vi "Chart.vi"() -> ()   [LabVIEW 2012]
uses:
  <vilib>/Utility/error.llb/DialogType.ctl
  <vilib>/Platform/TimedLoop/XDataNode/timing_clust.ctl
  <vilib>/Platform/TimedLoop/XDataNode/nitl_modes.ctl
  <vilib>/Platform/TimedLoop/XDataNode/wakeup.ctl
  <vilib>/Utility/error.llb/whitespace.ctl
  <vilib>/printing/EasyPrintingControls.llb/contents.ctl
  <vilib>/printing/EasyPrintingControls.llb/custom_contents_options.ctl
  <vilib>/printing/EasyPrintingControls.llb/list_which_controls.ctl
  <vilib>/printing/EasyPrintingControls.llb/layout_options.ctl
  <vilib>/printing/EasyPrintingControls.llb/orientation.ctl
  <vilib>/printing/EasyPrintingControls.llb/panel_scaling_for_page.ctl
  <vilib>/printing/EasyPrintingControls.llb/margins.ctl
  <vilib>/printing/EasyPrintingControls.llb/margin_values.ctl
  <vilib>/printing/EasyPrintingControls.llb/measurement_system.ctl
  <vilib>/printing/EasyPrintingControls.llb/printer_options.ctl
  <vilib>/printing/EasyPrintingControls.llb/printing_method.ctl
  <vilib>/printing/EasyPrintingControls.llb/color_or_monochrome.ctl
  <vilib>/printing/EasyPrintingControls.llb/page_header_options.ctl
  <vilib>/printing/EasyPrintingControls.llb/page_headers.ctl
  <vilib>/printing/EasyPrintingControls.llb/page_header_content_options.ctl
  <vilib>/DAQmx/read.llb/DAQmx Read (Analog 1D Wfm NChan NSamp).vi
  <vilib>/DAQmx/configure/timing.llb/DAQmx Timing (Sample Clock).vi
  <vilib>/DAQmx/create/channels.llb/DAQmx Create Channel (AI-Voltage-Basic).vi
  <vilib>/DAQmx/miscellaneous.llb/DAQmx Fill In Error Info.vi
  <vilib>/printing/EasyPrinting.llb/Easy Print VI Panel or Documentation (path).vi
  <vilib>/Platform/TimedLoop/XDataNode/XDataNode.xnode
  <vilib>/Platform/TimedLoop/XDataNode/XDNodeRunTimeDep.lvlib
  <resource>/objmgr/daqmx.rc
  <vilib>/Utility/NIReport.llb/NI_ReportGenerationCore.lvlib
panel:
  in  "Reset":bool
  in  "stop":bool
  in  "Tab Control":T1(tab)
  in  "Print1":bool
  in  "Capture1":bool
  in  "Samples Per Second":dbl(knob)=1.0 min=1.0 max=10.0 step=1.0 scale=1.0..10.0
  out "Waveform Chart1":waveform(dbl)(graph)
  in  "Clear1":bool
  in  "Save1":bool
  in  "Samples box1":bool
  in  "Title1":bool
  in  "Print12":bool
  out "Waveform Chart":dynamicdata(graph)
  in  "Capture12":bool
  in  "Clear12":bool
  in  "Save12":bool
  in  "Title12":bool
  in  "Samples Per Second":dbl(knob)=1.0 min=1.0 max=10.0 step=1.0 scale=1.0..10.0
  in  "Samples box12":bool
  in  "Print123":bool
  in  "Capture123":bool
  in  "Samples Per Second":dbl(knob)=1.0 min=1.0 max=10.0 step=1.0 scale=1.0..10.0
  out "Waveform Chart123":dynamicdata(graph)
  in  "Clear123":bool
  in  "Save123":bool
  in  "Samples box123":bool
  in  "Title123":bool
  in  "Print1234":bool
  in  "Capture1234":bool
  in  "Samples Per Second":dbl(knob)=1.0 min=1.0 max=10.0 step=1.0 scale=1.0..10.0
  in  "Save1234":bool
  in  "Samples box1234":bool
  in  "Title1234":bool
  out "Waveform Chart1234":dynamicdata(graph)
  in  "Clear1234":bool
  in  "Print1v2":bool
  out "XY Graph":cluster{"Y":dbl[], "Y":dbl[]}[](graph)
  in  "Title1v2":bool
  in  "Save1v2":bool
  in  "Clear1v2":bool
  in  "Samples Per Second":dbl(knob)=1.0 min=1.0 max=10.0 step=1.0 scale=1.0..10.0
  in  "Capture1v2":bool
  in  "Samples box1v2":bool
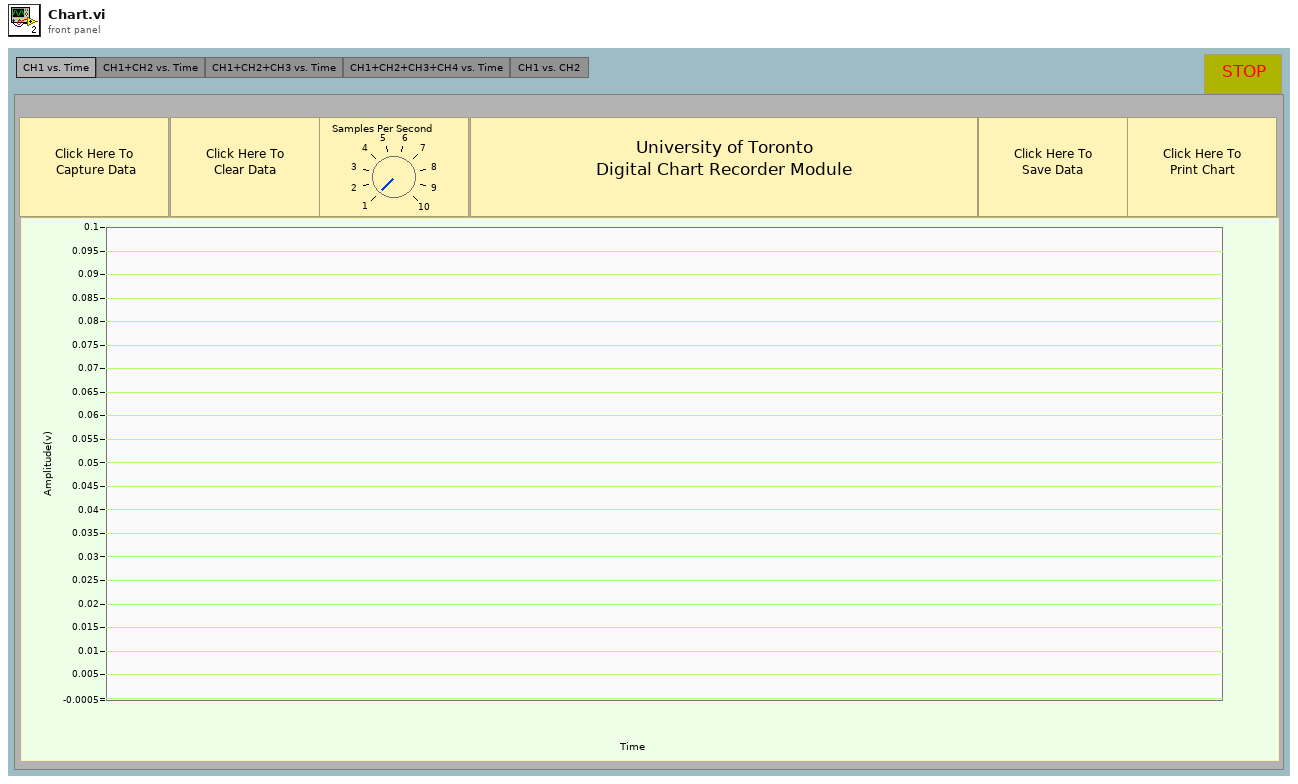
[diagram p1: front panel]
types:
  T1 = enum32{"CH1 vs. Time", "CH1+CH2 vs. Time", "CH1+CH2+CH3 vs. Time", "CH1+CH2+CH3+CH4 vs. Time", "CH1 vs. CH2 "}
  T2 = enum8{"Enabled", "Disabled", "Disabled and Grayed Out"}
  T3 = enum32{"CH1 vs. Time", "CH1+CH2 vs. Time", "CH1+CH2+CH3 vs. Time", "CH1+CH2+CH3+CH4 vs. Time", "CH1 vs. CH2  "}
  T4 = typedef "XDNodeRunTimeDep.lvlib/timing_clust.ctl" = cluster{"Expected End [f-1]":u64, "Actual End [f-1]":u64, "Finished Late? [f-1]":bool, "Expected End [i-1]":u64, "Actual End [i-1]":u64, "Finished Late? [i-1]":bool, "Expected Start [i]":u64, "Actual Start [i]":u64, "Expected Start [f]":u64, "Actual Start [f]":u64, "Source Name":string, "Structure Name":string, "Period":i64, "Deadline":i64, "Offset":i64, "Start":i64, "Priority":i32, "Timeout":i32, "Mode":T5, "Wakeup Reason":T6, "Error":errorcluster, "Source Type":string, "Secondary Source Type":string, "Global End Time":u64, "Global Start Time":u64, "Frame Duration":u64, "Iteration Duration":u64, "Assigned CPU":i32, "I/O Scan Engine Mode":u32}
  T5 = typedef "XDNodeRunTimeDep.lvlib/nitl_modes.ctl" = enum32{"No Change", "Process missed periods, maintain original phase", "Discard missed periods, maintain original phase", "Process missed periods, ignore original phase", "Discard missed periods, ignore original phase"}
  T6 = typedef "XDNodeRunTimeDep.lvlib/wakeup.ctl" = enum32{"Normal", "Aborted", "Asynchronous wakeup", "Timing source error", "Timed loop error", "Timeout"}
  T7 = enum16{"open", "replace", "create", "open or create", "replace or create", "replace or create with confirmation"}
  T8 = typedef "NI_ReportGenerationCore.lvlib/layout_options.ctl" = cluster{"orientation (unchanged)":T9, "panel scaling for page (unchanged)":T10, "margins":T11, "printer options":T14, "page header options":T17}
  T9 = typedef "NI_ReportGenerationCore.lvlib/orientation.ctl" = u16
  T10 = typedef "NI_ReportGenerationCore.lvlib/panel_scaling_for_page.ctl" = u16
  T11 = typedef "NI_ReportGenerationCore.lvlib/margins.ctl" = cluster{"override VI margins (false)":bool, "margins (1.00)":T12, "measurement system (default)":T13}
  T12 = typedef "NI_ReportGenerationCore.lvlib/margin_values.ctl" = cluster{"top":dbl, "left":dbl, "right":dbl, "bottom":dbl}
  T13 = typedef "NI_ReportGenerationCore.lvlib/measurement_system.ctl" = u16
  T14 = typedef "NI_ReportGenerationCore.lvlib/printer_options.ctl" = cluster{"destination printer name (current)":string, "printing method (unchanged)":T15, "color or monochrome (unchanged)":T16}
  T15 = typedef "NI_ReportGenerationCore.lvlib/printing_method.ctl" = u16
  T16 = typedef "NI_ReportGenerationCore.lvlib/color_or_monochrome.ctl" = u16
  T17 = typedef "NI_ReportGenerationCore.lvlib/page_header_options.ctl" = cluster{"page headers (unchanged)":T18, "page header content options":T19}
  T18 = typedef "NI_ReportGenerationCore.lvlib/page_headers.ctl" = u16
  T19 = typedef "NI_ReportGenerationCore.lvlib/page_header_content_options.ctl" = cluster{"Include VI Name":bool, "Include VI Path":bool, "Include Last Modification Date":bool, "Include Date Printed":bool, "Include Page Number":bool, "Include VI Icon":bool}
  T20 = typedef "NI_ReportGenerationCore.lvlib/custom_contents_options.ctl" = cluster{"include VI connector and icon":bool, "include VI description":bool, "include front panel":bool, "surround front panel with border":bool, "list of controls options":cluster{"include list of controls":bool, "list which controls?":T21, "include control descriptions?":bool, "include control data types?":bool}, "block diagram options":cluster{"include block diagram":bool, "hidden frames":bool, "ordered (repeat from higher level if nested)":bool}, "include VI hierarchy":bool, "include list of subVIs":bool, "include VI history":bool, "include Express VI configuration information":bool}
  T21 = typedef "NI_ReportGenerationCore.lvlib/list_which_controls.ctl" = u16
  T22 = typedef "DialogType.ctl" = u16
  T23 = typedef "whitespace.ctl" = u16
  T24 = typedef "NI_ReportGenerationCore.lvlib/contents.ctl" = u16
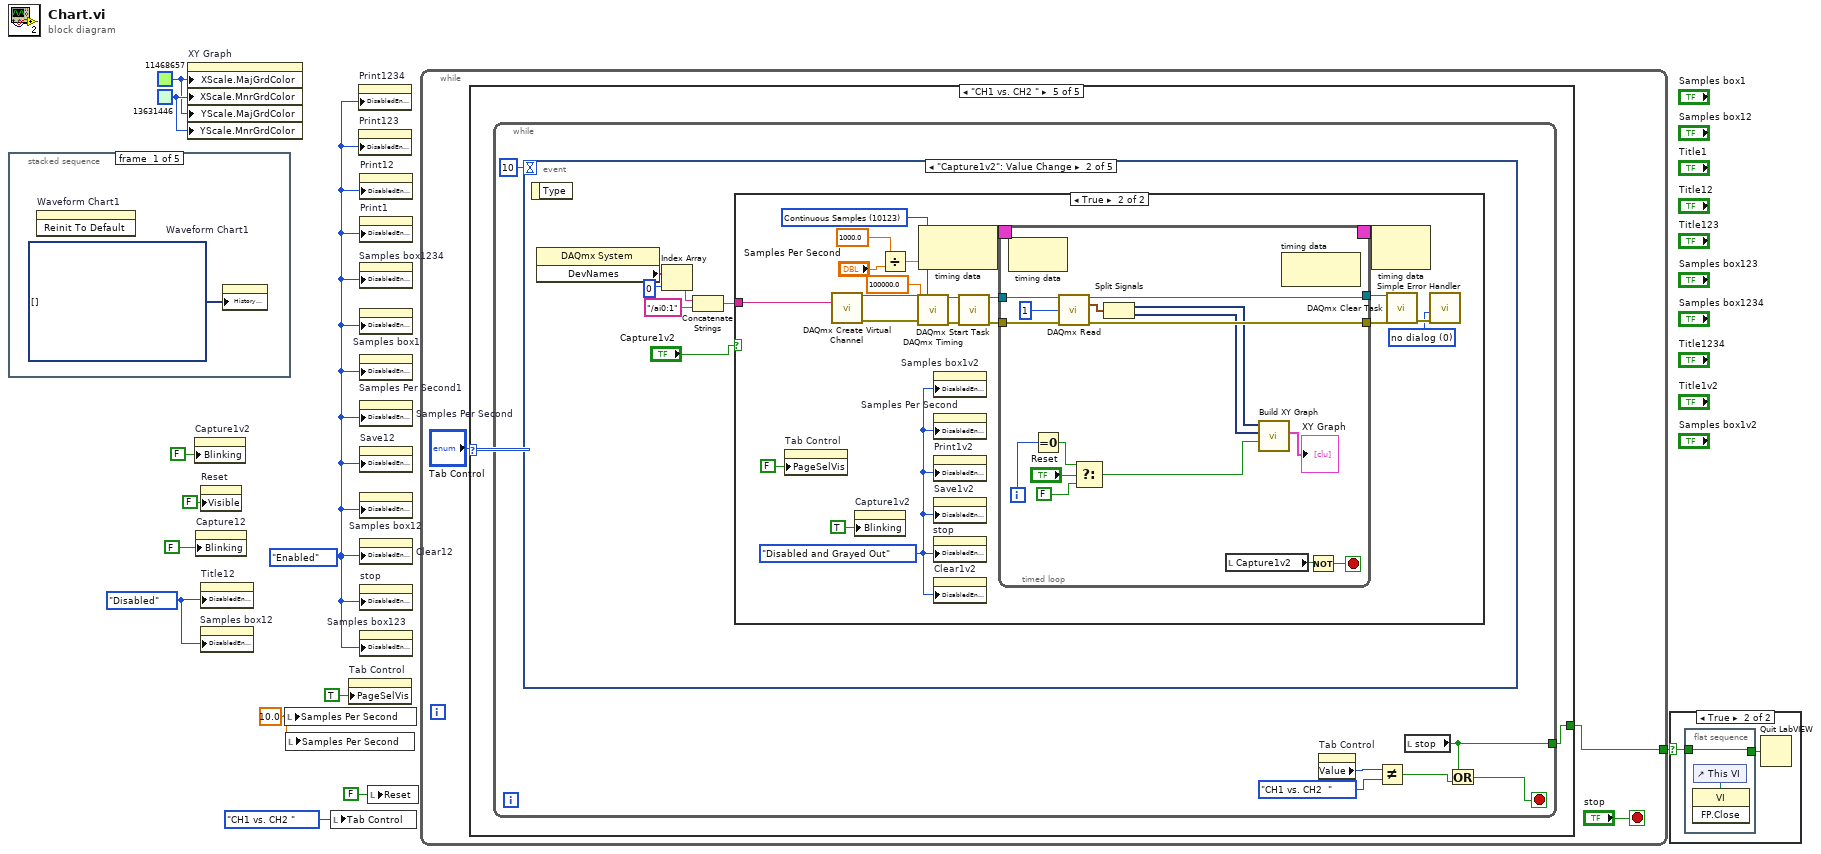
[diagram p0: block diagram]
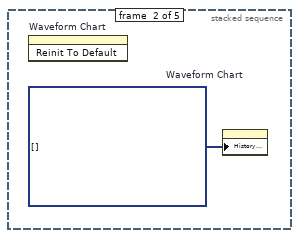
[diagram p2: hidden frame]
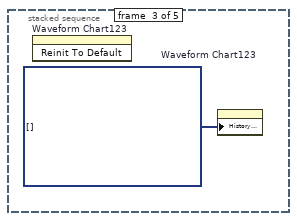
[diagram p3: hidden frame]
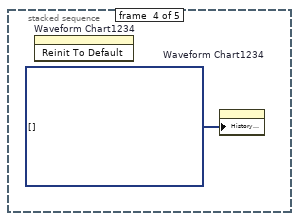
[diagram p4: hidden frame]
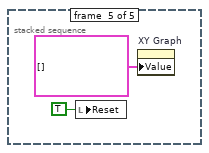
[diagram p5: hidden frame]
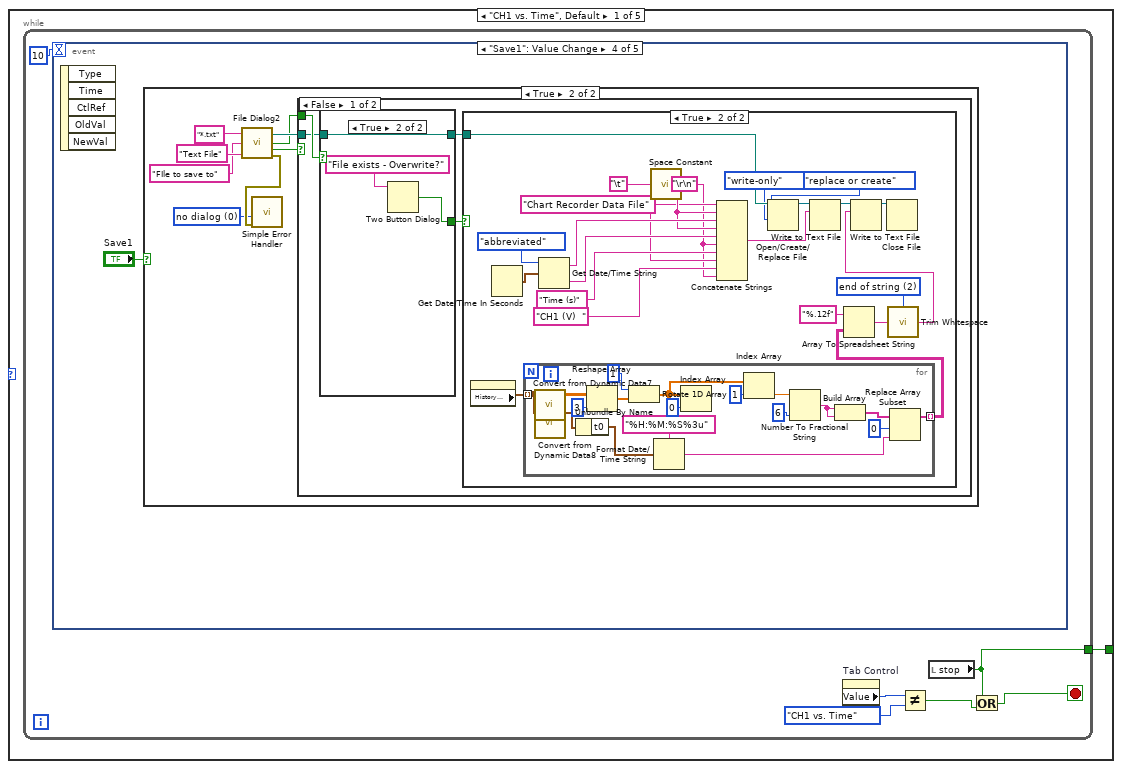
[diagram p7: hidden frame]
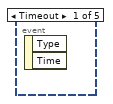
[diagram p8: hidden frame]
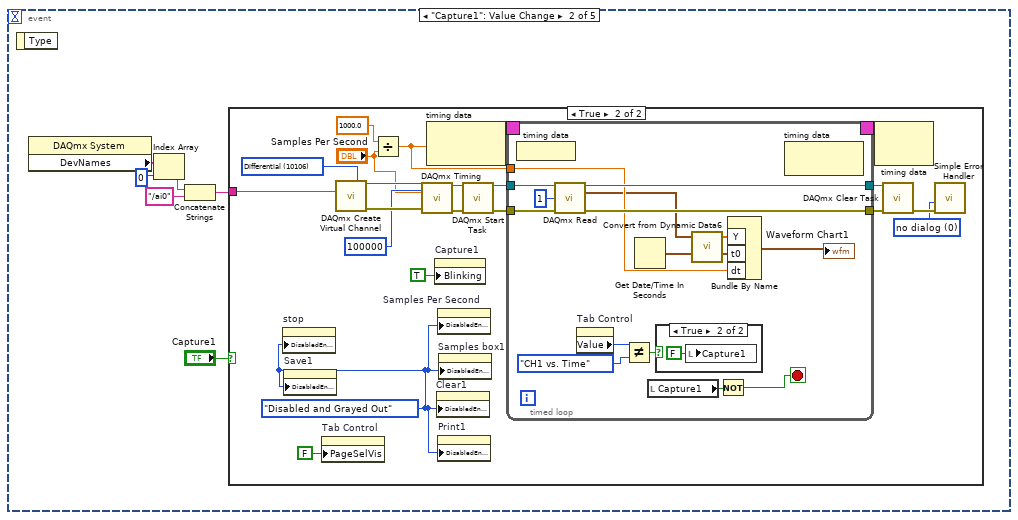
[diagram p9: hidden frame]
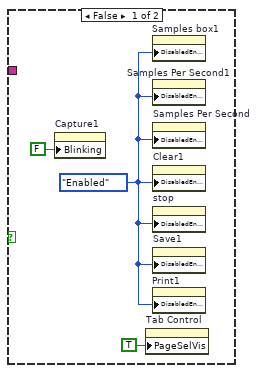
[diagram p10: hidden frame]
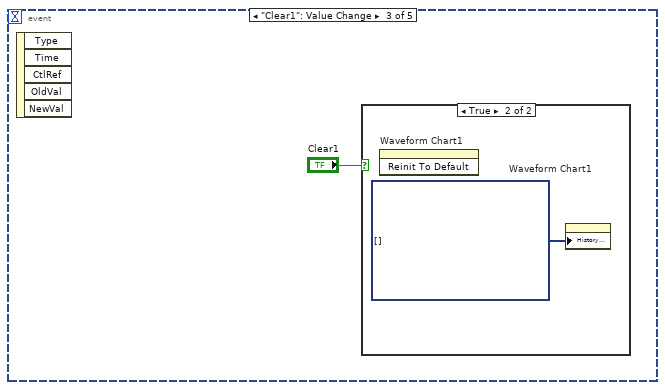
[diagram p12: hidden frame]
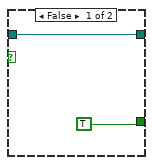
[diagram p16: hidden frame]
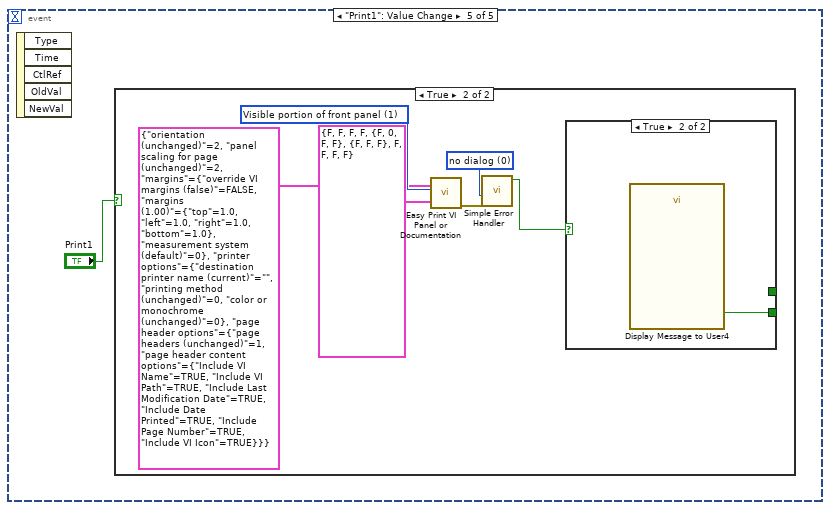
[diagram p18: hidden frame]
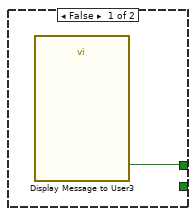
[diagram p20: hidden frame]
diagram:
  w1 = 10.0 ("Samples Per Second")
  w6 = u32 13631446
  w5 = u32 11468657
  w11 = T2."Disabled" ("Disabled")
  w4 = T2."Enabled" ("Disabled")
  n1 = stacked-sequence {
    frame #0 {
      n2 = invoke on="Waveform Chart1" class="WFChart (strict)" method="Reinit To Default"() -> ()  [unwired: 3 in, 3 out]
      n3 = property on="Waveform Chart1" class="WFChart (strict)"("History Data"=dynamicdata[] []) -> ()  [unwired: 2 in, 2 out]
    }
    frame #1 {
      n4 = invoke on="Waveform Chart" class="WFChart (strict)" method="Reinit To Default"() -> ()  [unwired: 3 in, 3 out]
      n5 = property on="Waveform Chart" class="WFChart (strict)"("History Data"=dynamicdata[] []) -> ()  [unwired: 2 in, 2 out]
    }
    frame #2 {
      n6 = invoke on="Waveform Chart123" class="WFChart (strict)" method="Reinit To Default"() -> ()  [unwired: 3 in, 3 out]
      n7 = property on="Waveform Chart123" class="WFChart (strict)"("History Data"=dynamicdata[] []) -> ()  [unwired: 2 in, 2 out]
    }
    frame #3 {
      n8 = invoke on="Waveform Chart1234" class="WFChart (strict)" method="Reinit To Default"() -> ()  [unwired: 3 in, 3 out]
      n9 = property on="Waveform Chart1234" class="WFChart (strict)"("History Data"=dynamicdata[] []) -> ()  [unwired: 2 in, 2 out]
    }
    frame #4 {
      n10 = local write "Reset"(TRUE ("Reset")) -> ()
      n11 = property on="XY Graph" class="XYGraph (strict)"("Value"=cluster{"Y":dbl[], "Y":dbl[]}[] [] ("XY Graph")) -> ()  [unwired: 2 in, 2 out]
    }
  }
  n12 = property on="XY Graph" class="XYGraph (strict)"("XScale.MajGrdColor"=w5, "XScale.MnrGrdColor"=w6, "YScale.MajGrdColor"=w5, "YScale.MnrGrdColor"=w6) -> ()  [unwired: 2 in, 2 out]
  n13 = property on="Capture1v2" class="Bool (strict)"("Blinking"=FALSE) -> ()  [unwired: 2 in, 2 out]
  n14 = property on="Capture12" class="Bool (strict)"("Blinking"=FALSE) -> ()  [unwired: 2 in, 2 out]
  n15 = property on="Reset" class="Bool (strict)"("Visible"=FALSE) -> ()  [unwired: 2 in, 2 out]
  n16 = property on="Title12" class="Bool"("DisabledEnum"=w11) -> ()  [unwired: 2 in, 2 out]
  n17 = property on="Samples box12" class="Bool"("DisabledEnum"=w11) -> ()  [unwired: 2 in, 2 out]
  n18 = local write "Samples Per Second"(w1) -> ()
  n19 = local write "Samples Per Second"(w1) -> ()
  n20 = local write "Tab Control"(T1."CH1 vs. CH2 " ("Tab Control")) -> ()
  n21 = property on="Tab Control" class="TabCtl (strict)"("PageSelVis"=TRUE ("Page Selector Visible")) -> ()  [unwired: 2 in, 2 out]
  n22 = property on="Print1234" class="Bool"("DisabledEnum"=w4) -> ()  [unwired: 2 in, 2 out]
  n23 = property on="Print123" class="Bool"("DisabledEnum"=w4) -> ()  [unwired: 2 in, 2 out]
  n24 = property on="Print12" class="Bool"("DisabledEnum"=w4) -> ()  [unwired: 2 in, 2 out]
  n25 = property on="Print1" class="Bool"("DisabledEnum"=w4) -> ()  [unwired: 2 in, 2 out]
  n26 = property on="Samples box1234" class="Bool"("DisabledEnum"=w4) -> ()  [unwired: 2 in, 2 out]
  n27 = property on="Samples box1" class="Bool"("DisabledEnum"=w4) -> ()  [unwired: 2 in, 2 out]
  n28 = property on="Samples Per Second1" class="Knob (strict)"("DisabledEnum"=w4) -> ()  [unwired: 2 in, 2 out]
  n29 = property on="Samples Per Second" class="Knob (strict)"("DisabledEnum"=w4) -> ()  [unwired: 2 in, 2 out]
  n30 = property on="Save12" class="Bool"("DisabledEnum"=w4) -> ()  [unwired: 2 in, 2 out]
  n31 = property on="Samples box12" class="Bool"("DisabledEnum"=w4) -> ()  [unwired: 2 in, 2 out]
  n32 = property on="Clear12" class="Bool"("DisabledEnum"=w4) -> ()  [unwired: 2 in, 2 out]
  n33 = property on="stop" class="Bool (strict)"("DisabledEnum"=w4) -> ()  [unwired: 2 in, 2 out]
  n34 = property on="Samples box123" class="Bool"("DisabledEnum"=w4) -> ()  [unwired: 2 in, 2 out]
  n35 = local write "Reset"(FALSE ("Reset")) -> ()
  n36 = while {
    tunnel: [w19] -> w10
    stop <- "stop" stop-if-true
    n37 = case shown="\"CH1 vs. CH2 \"" "Tab Control" {
      tunnel: [w22 w151 w285 w426 w574] -> w19
      frame "CH1 vs. Time", Default {
        n38 = while {
          tunnel: [w25] -> w22
          stop <- w23 stop-if-true
          n39 = event shown="[3] \"Save1\": Value Change" {
            selector: _ -> [_ _ _ _ _]
            dyn-events: _ -> [_ _ _ _ _]
            timeout: 10 -> [_ _ _ _ _]
            event Timeout {
              n40 = event-data() -> ()  [unwired: 1 in, 2 out]
            }
            event "Capture1": Value Change {
              n41 = event-data() -> ()  [unwired: 1 in, 1 out]
              n42 = property class="DAQmx System"() -> ("DevNames"=w31:tag[])  [unwired: 2 in, 2 out]
              n43 = Index Array(array=w31, index=0) -> (element=w34:tag)
              n44 = Concatenate Strings(w34, "/ai0" ("string")) -> (w30:string)
              n45 = case shown="True" "Capture1" {
                tunnel: w30 -> [_ w41]
                frame False {
                  w36 = T2."Enabled" ("Disabled")
                  n46 = property on="Capture1" class="Bool (strict)"("Blinking"=FALSE) -> ()  [unwired: 2 in, 2 out]
                  n47 = property on="Tab Control" class="TabCtl (strict)"("PageSelVis"=TRUE ("Page Selector Visible")) -> ()  [unwired: 2 in, 2 out]
                  n48 = property on="Samples box1" class="Bool"("DisabledEnum"=w36) -> ()  [unwired: 2 in, 2 out]
                  n49 = property on="Samples Per Second1" class="Knob (strict)"("DisabledEnum"=w36) -> ()  [unwired: 2 in, 2 out]
                  n50 = property on="Samples Per Second" class="Knob (strict)"("DisabledEnum"=w36) -> ()  [unwired: 2 in, 2 out]
                  n51 = property on="Clear1" class="Bool"("DisabledEnum"=w36) -> ()  [unwired: 2 in, 2 out]
                  n52 = property on="stop" class="Bool (strict)"("DisabledEnum"=w36) -> ()  [unwired: 2 in, 2 out]
                  n53 = property on="Save1" class="Bool"("DisabledEnum"=w36) -> ()  [unwired: 2 in, 2 out]
                  n54 = property on="Print1" class="Bool"("DisabledEnum"=w36) -> ()  [unwired: 2 in, 2 out]
                }
                frame True {
                  w39 = T2."Disabled and Grayed Out" ("Disabled")
                  w48 = 10106 items=["default"=-1, "RSE"=10083, "NRSE"=10078, "Differential"=10106, "Pseudodifferential"=12529] ("input terminal configuration")
                  w51 = T22 0 items=["no dialog", "OK message", "continue or stop message", "OK message + warnings", "continue/stop + warnings"] ("type of dialog (OK msg:1)")
                  n55 = property on="stop" class="Bool (strict)"("DisabledEnum"=w39) -> ()  [unwired: 2 in, 2 out]
                  n56 = property on="Save1" class="Bool"("DisabledEnum"=w39) -> ()  [unwired: 2 in, 2 out]
                  n57 = property on="Tab Control" class="TabCtl (strict)"("PageSelVis"=FALSE ("Page Selector Visible")) -> ()  [unwired: 2 in, 2 out]
                  n58 = call-poly <vilib>:"DAQmx Create Virtual Channel.vi"("input terminal configuration"=w48, "physical channels"=w41) -> ("task out"=w58:refnum<k21>, "error out"=w56:errorcluster)  [unwired: 12 in]
                  n59 = Divide(x=1000.0, y="Samples Per Second") -> (x/y=w40:dbl)
                  n60 = call-poly <vilib>:"DAQmx Timing.vi"("task/channels in"=w58, "samples per channel"=100000, "rate"="Samples Per Second", "error in"=w56) -> ("task out"=w57:refnum<k21>, "error out"=w55:errorcluster)  [unwired: 10 in]
                  n61 = node-c288(w40) -> (w46:T4)
                  n62 = property on="Capture1" class="Bool (strict)"("Blinking"=TRUE) -> ()  [unwired: 2 in, 2 out]
                  n63 = property on="Clear1" class="Bool"("DisabledEnum"=w39) -> ()  [unwired: 2 in, 2 out]
                  n64 = property on="Samples Per Second" class="Knob (strict)"("DisabledEnum"=w39) -> ()  [unwired: 2 in, 2 out]
                  n65 = property on="Print1" class="Bool"("DisabledEnum"=w39) -> ()  [unwired: 2 in, 2 out]
                  n66 = property on="Samples box1" class="Bool"("DisabledEnum"=w39) -> ()  [unwired: 2 in, 2 out]
                  n67 = call <vilib>:"DAQmx Start Task.vi"("task/channels in"=w57, "error in"=w55) -> ("task out"=w54:refnum<k21>, "error out"=w53:errorcluster)  [unwired: 12 in]
                  n68 = timed-loop {
                    tunnel: w54 -> [w73]
                    tunnel: w53 -> [w72]
                    tunnel: [w71] -> w50
                    tunnel: [w70] -> w49
                    timing: w46 -> [_]
                    timing-out: [_] -> w45
                    tunnel: w40 -> [w67]
                    stop <- w60 stop-if-true
                    n69 = node-c288() -> ()  [unwired: 1 in]
                    n70 = call-poly <vilib>:"DAQmx Read.vi"("task/channels in"=w73, "number of samples per channel"=1, "error in"=w72) -> ("task out"=w71:refnum<k21>, "data"=w63:waveform(dbl)[], "error out"=w70:errorcluster)  [unwired: 10 in]
                    n71 = property on="Tab Control" class="TabCtl (strict)"() -> ("Value"=w61:T1)  [unwired: 2 in, 2 out]
                    n72 = Not Equal?(x=w61, y=T1."CH1 vs. Time" ("Tab Control")) -> (x != y?=w59:bool)
                    n73 = Get Date/Time In Seconds() -> (seconds since 1Jan1904=w66:timestamp)
                    n74 = local read "Capture1"() -> (w65:bool)
                    n75 = case shown="True" w59 {
                      frame False {
                      }
                      frame True {
                        n76 = local write "Capture1"(FALSE ("Capture1")) -> ()
                      }
                    }
                    n77 = call "Convert from Dynamic Data6"("Dynamic Data Type"=w63) -> ("Array"=w68:dbl[])  [unwired: 3 in]
                    n78 = Not(x=w65) -> (.not. x?=w60:bool)
                    n79 = Bundle By Name("Y"=w68, "t0"=w66, "dt"=w67) -> (→"Waveform Chart1":waveform(dbl))  [unwired: 1 in]
                    n80 = node-c288() -> ()  [unwired: 1 in, 1 out]
                  }
                  n81 = node-c288(w45) -> ()  [unwired: 1 out]
                  n82 = call <vilib>:"DAQmx Clear Task.vi"("task in"=w50, "error in"=w49) -> ("error out"=w52:errorcluster)  [unwired: 13 in]
                  n83 = call <vilib>:"Simple Error Handler.vi"("type of dialog (OK msg:1)"=w51, "error in (no error)"=w52) -> ()  [unwired: 3 in, 5 out]
                }
              }
            }
            event "Clear1": Value Change {
              n84 = event-data() -> ()  [unwired: 1 in, 5 out]
              n85 = case shown="True" "Clear1" {
                frame False {
                }
                frame True {
                  n86 = invoke on="Waveform Chart1" class="WFChart (strict)" method="Reinit To Default"() -> ()  [unwired: 3 in, 3 out]
                  n87 = property on="Waveform Chart1" class="WFChart (strict)"("History Data"=dynamicdata[] []) -> ()  [unwired: 2 in, 2 out]
                }
              }
            }
            event "Save1": Value Change {
              n88 = event-data() -> ()  [unwired: 1 in, 5 out]
              n89 = case shown="True" "Save1" {
                frame False {
                }
                frame True {
                  w84 = T22 0 items=["no dialog", "OK message", "continue or stop message", "OK message + warnings", "continue/stop + warnings"] ("type of dialog (OK msg:1)")
                  n90 = call "File Dialog2"("prompt"="FIle to save to", "pattern (all files)"="*.txt", "pattern label"="Text File") -> ("selected path"=w88:path, "exists"=w86:bool, "cancelled"=w87:bool, "error out"=w85:errorcluster)  [unwired: 9 in]
                  n91 = call <vilib>:"Simple Error Handler.vi"("type of dialog (OK msg:1)"=w84, "error in (no error)"=w85) -> ()  [unwired: 3 in, 5 out]
                  n92 = case shown="False" w87 {
                    tunnel: w88 -> [w94 _]
                    tunnel: w86 -> [w95 _]
                    frame False {
                      n93 = case shown="True" w95 {
                        tunnel: w94 -> [w137 w140]
                        tunnel: [TRUE w139] -> w93
                        tunnel: [w137 w140] -> w92
                        frame False {
                        }
                        frame True {
                          n94 = Two Button Dialog(message="File exists - Overwrite?") -> (T button?=w139:bool)  [unwired: 2 in]
                        }
                      }
                      n95 = case shown="True" w93 {
                        tunnel: w92 -> [_ w118]
                        frame False {
                        }
                        frame True {
                          w105 = T23 2 items=["both", "start of string", "end of string"] ("location (both)")
                          w96 = "\r\n"
                          n96 = property on="Waveform Chart1" class="WFChart (strict)"() -> ("History Data"=w101:waveform(dbl)[])  [unwired: 2 in, 2 out]
                          n97 = Get Date/Time In Seconds() -> (seconds since 1Jan1904=w109:timestamp)
                          n98 = for {
                            tunnel: w101 -> [w121] mode=indexing
                            tunnel: [w124] -> w97 mode=indexing
                            n99 = call "Convert from Dynamic Data7"("Dynamic Data Type"=w121) -> ("Array"=w123:dbl[][])  [unwired: 3 in]
                            n100 = call "Convert from Dynamic Data8"("Dynamic Data Type"=w121) -> ("Waveform"=w120:waveform(dbl))  [unwired: 3 in]
                            n101 = Unbundle By Name(w120) -> ("t0"=w119:timestamp)
                            n102 = Reshape Array(w123, 3 ("dimension size")) -> (w135:dbl[])
                            n103 = Rotate 1D Array(1:w135, 2:1 ("n")) -> (0:w130:dbl[])
                            n104 = Format Date/Time String(time format string (%c)="%H:%M:%S%3u", seconds (now)=w119) -> (date/time string=w122:string)  [unwired: 1 in]
                            n105 = Index Array(array=w130, index=0) -> ()  [unwired: 1 out]
                            n106 = Index Array(array=w130, index=1) -> (element=w129:dbl)
                            n107 = Number To Fractional String(number=w129, precision (6)=i16 6 ("width (-)")) -> (F-format string=w127:string)  [unwired: 2 in]
                            n108 = Build Array(w127, w127) -> (w126:string[])
                            n109 = Replace Array Subset(array=w126, new element=w122, index=0) -> (w124:string[])
                          }
                          n110 = Get Date/Time String(date format (0)=enum16{"short", "long", "abbreviated"}."abbreviated", seconds (now)=w109) -> (date string=w111:string, time string=w112:string)  [unwired: 1 in]
                          n111 = call <vilib>:"Space Constant.vi"() -> ("String"=w106:string)
                          n112 = Concatenate Strings("Chart Recorder Data File" ("HeaderTxtIn"), w106, w111, w106, w112, w96, "Time (s)", "\t", "CH1 (V)  ", w96) -> (w103:string)
                          n113 = Open/Create/Replace File(file path (use dialog)=w118, operation (0:open)=T7."replace or create", access (0:read/write)=enum16{"read/write", "read-only", "write-only"}."write-only") -> (refnum out=w117:refnum<file>)  [unwired: 3 in, 2 out]
                          n114 = Write to Text File(file (use dialog)=w117, text=w103) -> (refnum out=w113:refnum<file>)  [unwired: 2 in, 2 out]
                          n115 = Array To Spreadsheet String(array=w97, 3:"%.12f" ("format string")) -> (spreadsheet string=w99:string)  [unwired: 1 in]
                          n116 = call <vilib>:"Trim Whitespace.vi"("string"=w99, "location (both)"=w105) -> ("trimmed string"=w104:string)
                          n117 = Write to Text File(file (use dialog)=w113, text=w104) -> (refnum out=w114:refnum<file>)  [unwired: 2 in, 2 out]
                          n118 = Close File(refnum=w114) -> ()  [unwired: 1 in, 2 out]
                        }
                      }
                    }
                    frame True {
                    }
                  }
                }
              }
            }
            event "Print1": Value Change {
              n119 = event-data() -> ()  [unwired: 1 in, 5 out]
              n120 = case shown="True" "Print1" {
                frame False {
                }
                frame True {
                  w144 = T22 0 items=["no dialog", "OK message", "continue or stop message", "OK message + warnings", "continue/stop + warnings"] ("type of dialog (OK msg:1)")
                  w148 = T24 1 items=["Complete front panel", "Visible portion of front panel", "Icon, description, panel and diagram", "Documentation: Using the panel", "Documentation: Using as a subVI", "Documentation: Complete", "Documentation: Custom"] ("contents (complete front panel)")
                  n121 = call-poly <vilib>:"Easy Print VI Panel or Documentation.vi"("custom contents options"=T20 {"include VI connector and icon"=FALSE, "include VI description"=FALSE, "include front panel"=FALSE, "surround front panel with border"=FALSE, "list of controls options"={"include list of controls"=FALSE, "list which controls?"=0, "include control descriptions?"=FALSE, "include control data types?"=FALSE}, "block diagram options"={"include block diagram"=FALSE, "hidden frames"=FALSE, "ordered (repeat from higher level if nested)"=FALSE}, "include VI hierarchy"=FALSE, "include list of subVIs"=FALSE, "include VI history"=FALSE, "include Express VI configuration information"=FALSE}, "layout options"=T8 {"orientation (unchanged)"=2, "panel scaling for page (unchanged)"=2, "margins"={"override VI margins (false)"=FALSE, "margins (1.00)"={"top"=1.0, "left"=1.0, "right"=1.0, "bottom"=1.0}, "measurement system (default)"=0}, "printer options"={"destination printer name (current)"="", "printing method (unchanged)"=0, "color or monochrome (unchanged)"=0}, "page header options"={"page headers (unchanged)"=1, "page header content options"={"Include VI Name"=TRUE, "Include VI Path"=TRUE, "Include Last Modification Date"=TRUE, "Include Date Printed"=TRUE, "Include Page Number"=TRUE, "Include VI Icon"=TRUE}}}, "contents (complete front panel)"=w148) -> ("error out"=w145:errorcluster)  [unwired: 3 in, 5 out]
                  n122 = call <vilib>:"Simple Error Handler.vi"("type of dialog (OK msg:1)"=w144, "error in (no error)"=w145) -> ("error?"=w143:bool)  [unwired: 3 in, 4 out]
                  n123 = case shown="True" w143 {
                    tunnel: [w149 _] -> _
                    tunnel: [_ w150] -> _
                    frame False {
                      n124 = call "Display Message to User3"() -> ("OK"=w149:bool)  [unwired: 10 in, 1 out]
                    }
                    frame True {
                      n125 = call "Display Message to User4"() -> ("OK"=w150:bool)  [unwired: 10 in, 1 out]
                    }
                  }
                }
              }
            }
          }
          n126 = property on="Tab Control" class="TabCtl (strict)"() -> ("Value"=w26:T1)  [unwired: 2 in, 2 out]
          n127 = Not Equal?(x=w26, y=T3."CH1 vs. Time" ("Tab Control")) -> (x != y?=w24:bool)
          n128 = local read "stop"() -> (w25:bool)
          n129 = Or(x=w25, y=w24) -> (x .or. y?=w23:bool)
        }
      }
      frame "CH1+CH2 vs. Time" {
        n130 = while {
          tunnel: [w152] -> w151
          stop <- w153 stop-if-true
          n131 = event shown="[1] \"Capture12\": Value Change" {
            selector: _ -> [_ _ _ _ _]
            dyn-events: _ -> [_ _ _ _ _]
            timeout: 10 -> [_ _ _ _ _]
            event Timeout {
              n132 = event-data() -> ()  [unwired: 1 in, 2 out]
            }
            event "Capture12": Value Change {
              n133 = event-data() -> ()  [unwired: 1 in, 1 out]
              n134 = property class="DAQmx System"() -> ("DevNames"=w160:tag[])  [unwired: 2 in, 2 out]
              n135 = Index Array(array=w160, index=0) -> (element=w163:tag)
              n136 = Concatenate Strings(w163, "/ai0:1" ("string")) -> (w159:string)
              n137 = case shown="True" "Capture12" {
                tunnel: w159 -> [_ w170]
                frame False {
                  w165 = T2."Enabled" ("Disabled")
                  n138 = property on="Capture12" class="Bool (strict)"("Blinking"=FALSE) -> ()  [unwired: 2 in, 2 out]
                  n139 = property on="Tab Control" class="TabCtl (strict)"("PageSelVis"=TRUE ("Page Selector Visible")) -> ()  [unwired: 2 in, 2 out]
                  n140 = property on="Samples box12" class="Bool"("DisabledEnum"=w165) -> ()  [unwired: 2 in, 2 out]
                  n141 = property on="Samples Per Second" class="Knob (strict)"("DisabledEnum"=w165) -> ()  [unwired: 2 in, 2 out]
                  n142 = property on="Clear12" class="Bool"("DisabledEnum"=w165) -> ()  [unwired: 2 in, 2 out]
                  n143 = property on="stop" class="Bool (strict)"("DisabledEnum"=w165) -> ()  [unwired: 2 in, 2 out]
                  n144 = property on="Save12" class="Bool"("DisabledEnum"=w165) -> ()  [unwired: 2 in, 2 out]
                  n145 = property on="Print12" class="Bool"("DisabledEnum"=w165) -> ()  [unwired: 2 in, 2 out]
                }
                frame True {
                  w168 = T2."Disabled and Grayed Out" ("Disabled")
                  w177 = 10106 items=["default"=-1, "RSE"=10083, "NRSE"=10078, "Differential"=10106, "Pseudodifferential"=12529] ("input terminal configuration")
                  w180 = T22 0 items=["no dialog", "OK message", "continue or stop message", "OK message + warnings", "continue/stop + warnings"] ("type of dialog (OK msg:1)")
                  n146 = call-poly <vilib>:"DAQmx Create Virtual Channel.vi"("input terminal configuration"=w177, "physical channels"=w170) -> ("task out"=w187:refnum<k21>, "error out"=w185:errorcluster)  [unwired: 12 in]
                  n147 = property on="Tab Control" class="TabCtl (strict)"("PageSelVis"=FALSE ("Page Selector Visible")) -> ()  [unwired: 2 in, 2 out]
                  n148 = property on="Capture12" class="Bool (strict)"("Blinking"=TRUE) -> ()  [unwired: 2 in, 2 out]
                  n149 = Divide(x=1000.0, y="Samples Per Second") -> (x/y=w169:dbl)
                  n150 = call-poly <vilib>:"DAQmx Timing.vi"("task/channels in"=w187, "samples per channel"=100000, "rate"="Samples Per Second", "error in"=w185) -> ("task out"=w186:refnum<k21>, "error out"=w184:errorcluster)  [unwired: 10 in]
                  n151 = node-c288(w169) -> (w175:T4)
                  n152 = property on="Samples Per Second" class="Knob (strict)"("DisabledEnum"=w168) -> ()  [unwired: 2 in, 2 out]
                  n153 = property on="stop" class="Bool (strict)"("DisabledEnum"=w168) -> ()  [unwired: 2 in, 2 out]
                  n154 = property on="Clear12" class="Bool"("DisabledEnum"=w168) -> ()  [unwired: 2 in, 2 out]
                  n155 = property on="Save12" class="Bool"("DisabledEnum"=w168) -> ()  [unwired: 2 in, 2 out]
                  n156 = property on="Samples box12" class="Bool"("DisabledEnum"=w168) -> ()  [unwired: 2 in, 2 out]
                  n157 = property on="Print12" class="Bool"("DisabledEnum"=w168) -> ()  [unwired: 2 in, 2 out]
                  n158 = call <vilib>:"DAQmx Start Task.vi"("task/channels in"=w186, "error in"=w184) -> ("task out"=w183:refnum<k21>, "error out"=w182:errorcluster)  [unwired: 12 in]
                  n159 = timed-loop {
                    tunnel: w183 -> [w204]
                    tunnel: w182 -> [w203]
                    tunnel: [w202] -> w179
                    tunnel: [w201] -> w178
                    timing: w175 -> [_]
                    timing-out: [_] -> w174
                    tunnel: w169 -> [w192]
                    stop <- w193 stop-if-true
                    n160 = node-c288() -> ()  [unwired: 1 in]
                    n161 = call-poly <vilib>:"DAQmx Read.vi"("task/channels in"=w204, "number of samples per channel"=1, "error in"=w203) -> ("task out"=w202:refnum<k21>, "data"=w199:waveform(dbl)[], "error out"=w201:errorcluster)  [unwired: 10 in]
                    n162 = Split Signals(w199) -> (w196:dynamicdata, w198:dynamicdata)  [unwired: 2 in]
                    n163 = Get Date/Time In Seconds() -> (seconds since 1Jan1904=w189:timestamp)
                    n164 = call "Convert from Dynamic Data"("Dynamic Data Type"=w196) -> ("Array"=w195:dbl[])  [unwired: 3 in]
                    n165 = call "Convert from Dynamic Data2"("Dynamic Data Type"=w198) -> ("Array"=w197:dbl[])  [unwired: 3 in]
                    n166 = Bundle By Name("Y"=w195, "t0"=w189, "dt"=w192) -> (w194:waveform(dbl))  [unwired: 1 in]
                    n167 = Bundle By Name("Y"=w197, "t0"=w189, "dt"=w192) -> (w191:waveform(dbl))  [unwired: 1 in]
                    n168 = local read "Capture12"() -> (w188:bool)
                    n169 = Merge Signals(w194, w191) -> (→"Waveform Chart":dynamicdata)
                    n170 = node-c288() -> ()  [unwired: 1 in, 1 out]
                    n171 = Not(x=w188) -> (.not. x?=w193:bool)
                  }
                  n172 = node-c288(w174) -> ()  [unwired: 1 out]
                  n173 = call <vilib>:"DAQmx Clear Task.vi"("task in"=w179, "error in"=w178) -> ("error out"=w181:errorcluster)  [unwired: 13 in]
                  n174 = call <vilib>:"Simple Error Handler.vi"("type of dialog (OK msg:1)"=w180, "error in (no error)"=w181) -> ()  [unwired: 3 in, 5 out]
                }
              }
            }
            event "Clear12": Value Change {
              n175 = event-data() -> ()  [unwired: 1 in, 5 out]
              n176 = case shown="True" "Clear12" {
                frame False {
                }
                frame True {
                  n177 = invoke on="Waveform Chart" class="WFChart (strict)" method="Reinit To Default"() -> ()  [unwired: 3 in, 3 out]
                  n178 = property on="Waveform Chart" class="WFChart (strict)"("History Data"=dynamicdata[] []) -> ()  [unwired: 2 in, 2 out]
                }
              }
            }
            event "Save12": Value Change {
              n179 = event-data() -> ()  [unwired: 1 in, 5 out]
              n180 = case shown="True" "Save12" {
                frame False {
                }
                frame True {
                  w214 = T22 0 items=["no dialog", "OK message", "continue or stop message", "OK message + warnings", "continue/stop + warnings"] ("type of dialog (OK msg:1)")
                  n181 = call "File Dialog"("prompt"="FIle to save to", "pattern (all files)"="*.txt", "pattern label"="Text File") -> ("selected path"=w218:path, "exists"=w216:bool, "cancelled"=w217:bool, "error out"=w215:errorcluster)  [unwired: 9 in]
                  n182 = call <vilib>:"Simple Error Handler.vi"("type of dialog (OK msg:1)"=w214, "error in (no error)"=w215) -> ()  [unwired: 3 in, 5 out]
                  n183 = case shown="False" w217 {
                    tunnel: w218 -> [w224 _]
                    tunnel: w216 -> [w225 _]
                    frame False {
                      n184 = case shown="True" w225 {
                        tunnel: w224 -> [w271 w274]
                        tunnel: [TRUE w273] -> w223
                        tunnel: [w271 w274] -> w222
                        frame False {
                        }
                        frame True {
                          n185 = Two Button Dialog(message="File exists - Overwrite?") -> (T button?=w273:bool)  [unwired: 2 in]
                        }
                      }
                      n186 = case shown="True" w223 {
                        tunnel: w222 -> [_ w249]
                        frame False {
                        }
                        frame True {
                          w229 = "\t"
                          w236 = T23 2 items=["both", "start of string", "end of string"] ("location (both)")
                          w230 = "\r\n"
                          n187 = property on="Waveform Chart" class="WFChart (strict)"() -> ("History Data"=w232:dynamicdata[])  [unwired: 2 in, 2 out]
                          n188 = Get Date/Time In Seconds() -> (seconds since 1Jan1904=w240:timestamp)
                          n189 = for {
                            tunnel: w232 -> [w252] mode=indexing
                            tunnel: [w255] -> w226 mode=indexing
                            w260 = i16 6 ("width (-)")
                            n190 = call "Convert from Dynamic Data3"("Dynamic Data Type"=w252) -> ("Array"=w254:dbl[][])  [unwired: 3 in]
                            n191 = call "Convert from Dynamic Data4"("Dynamic Data Type"=w252) -> ("Waveform"=w251:waveform(dbl))  [unwired: 3 in]
                            n192 = Unbundle By Name(w251) -> ("t0"=w250:timestamp)
                            n193 = Reshape Array(w254, 3 ("dimension size")) -> (w269:dbl[])
                            n194 = Rotate 1D Array(1:w269, 2:1 ("n")) -> (0:w263:dbl[])
                            n195 = Format Date/Time String(time format string (%c)="%H:%M:%S%3u", seconds (now)=w250) -> (date/time string=w253:string)  [unwired: 1 in]
                            n196 = Index Array(array=w263, index=0) -> ()  [unwired: 1 out]
                            n197 = Index Array(array=w263, index=1) -> (element=w262:dbl)
                            n198 = Index Array(array=w263, index=2) -> (element=w261:dbl)
                            n199 = Number To Fractional String(number=w262, precision (6)=w260) -> (F-format string=w258:string)  [unwired: 2 in]
                            n200 = Number To Fractional String(number=w261, precision (6)=w260) -> (F-format string=w259:string)  [unwired: 2 in]
                            n201 = Build Array(w258, w258, w259) -> (w257:string[])
                            n202 = Replace Array Subset(array=w257, new element=w253, index=0) -> (w255:string[])
                          }
                          n203 = Get Date/Time String(date format (0)=enum16{"short", "long", "abbreviated"}."abbreviated", seconds (now)=w240) -> (date string=w242:string, time string=w243:string)  [unwired: 1 in]
                          n204 = call <vilib>:"Space Constant.vi"() -> ("String"=w237:string)
                          n205 = Concatenate Strings("Chart Recorder Data File" ("HeaderTxtIn"), w237, w242, w237, w243, w230, "Time (s)", w229, "CH1 (V)  ", w229, "CH2 (V)  ", w230) -> (w234:string)
                          n206 = Open/Create/Replace File(file path (use dialog)=w249, operation (0:open)=T7."replace or create", access (0:read/write)=enum16{"read/write", "read-only", "write-only"}."write-only") -> (refnum out=w248:refnum<file>)  [unwired: 3 in, 2 out]
                          n207 = Write to Text File(file (use dialog)=w248, text=w234) -> (refnum out=w244:refnum<file>)  [unwired: 2 in, 2 out]
                          n208 = Array To Spreadsheet String(array=w226, 3:"%.12f" ("format string")) -> (spreadsheet string=w228:string)  [unwired: 1 in]
                          n209 = call <vilib>:"Trim Whitespace.vi"("string"=w228, "location (both)"=w236) -> ("trimmed string"=w235:string)
                          n210 = Write to Text File(file (use dialog)=w244, text=w235) -> (refnum out=w245:refnum<file>)  [unwired: 2 in, 2 out]
                          n211 = Close File(refnum=w245) -> ()  [unwired: 1 in, 2 out]
                        }
                      }
                    }
                    frame True {
                    }
                  }
                }
              }
            }
            event "Print12": Value Change {
              n212 = event-data() -> ()  [unwired: 1 in, 5 out]
              n213 = case shown="True" "Print12" {
                frame False {
                }
                frame True {
                  w278 = T22 0 items=["no dialog", "OK message", "continue or stop message", "OK message + warnings", "continue/stop + warnings"] ("type of dialog (OK msg:1)")
                  w282 = T24 1 items=["Complete front panel", "Visible portion of front panel", "Icon, description, panel and diagram", "Documentation: Using the panel", "Documentation: Using as a subVI", "Documentation: Complete", "Documentation: Custom"] ("contents (complete front panel)")
                  n214 = call-poly <vilib>:"Easy Print VI Panel or Documentation.vi"("custom contents options"=T20 {"include VI connector and icon"=FALSE, "include VI description"=FALSE, "include front panel"=FALSE, "surround front panel with border"=FALSE, "list of controls options"={"include list of controls"=FALSE, "list which controls?"=0, "include control descriptions?"=FALSE, "include control data types?"=FALSE}, "block diagram options"={"include block diagram"=FALSE, "hidden frames"=FALSE, "ordered (repeat from higher level if nested)"=FALSE}, "include VI hierarchy"=FALSE, "include list of subVIs"=FALSE, "include VI history"=FALSE, "include Express VI configuration information"=FALSE}, "layout options"=T8 {"orientation (unchanged)"=2, "panel scaling for page (unchanged)"=2, "margins"={"override VI margins (false)"=FALSE, "margins (1.00)"={"top"=1.0, "left"=1.0, "right"=1.0, "bottom"=1.0}, "measurement system (default)"=0}, "printer options"={"destination printer name (current)"="", "printing method (unchanged)"=0, "color or monochrome (unchanged)"=0}, "page header options"={"page headers (unchanged)"=1, "page header content options"={"Include VI Name"=TRUE, "Include VI Path"=TRUE, "Include Last Modification Date"=TRUE, "Include Date Printed"=TRUE, "Include Page Number"=TRUE, "Include VI Icon"=TRUE}}}, "contents (complete front panel)"=w282) -> ("error out"=w279:errorcluster)  [unwired: 3 in, 5 out]
                  n215 = call <vilib>:"Simple Error Handler.vi"("type of dialog (OK msg:1)"=w278, "error in (no error)"=w279) -> ("error?"=w277:bool)  [unwired: 3 in, 4 out]
                  n216 = case shown="True" w277 {
                    tunnel: [w283 _] -> _
                    tunnel: [_ w284] -> _
                    frame False {
                      n217 = call "Display Message to User5"() -> ("OK"=w283:bool)  [unwired: 10 in, 1 out]
                    }
                    frame True {
                      n218 = call "Display Message to User6"() -> ("OK"=w284:bool)  [unwired: 10 in, 1 out]
                    }
                  }
                }
              }
            }
          }
          n219 = property on="Tab Control" class="TabCtl (strict)"() -> ("Value"=w156:T1)  [unwired: 2 in, 2 out]
          n220 = local read "stop"() -> (w152:bool)
          n221 = Not Equal?(x=w156, y=T3."CH1+CH2 vs. Time" ("Tab Control")) -> (x != y?=w154:bool)
          n222 = Or(x=w152, y=w154) -> (x .or. y?=w153:bool)
        }
      }
      frame "CH1+CH2+CH3 vs. Time" {
        n223 = while {
          tunnel: [w286] -> w285
          stop <- w287 stop-if-true
          n224 = event shown="[2] \"Print123\": Value Change" {
            selector: _ -> [_ _ _ _ _]
            dyn-events: _ -> [_ _ _ _ _]
            timeout: 10 -> [_ _ _ _ _]
            event Timeout {
              n225 = event-data() -> ()  [unwired: 1 in, 2 out]
            }
            event "Capture123": Value Change {
              n226 = event-data() -> ()  [unwired: 1 in, 1 out]
              n227 = property class="DAQmx System"() -> ("DevNames"=w294:tag[])  [unwired: 2 in, 2 out]
              n228 = Index Array(array=w294, index=0) -> (element=w297:tag)
              n229 = Concatenate Strings(w297, "/ai0:2" ("string")) -> (w293:string)
              n230 = case shown="True" "Capture123" {
                tunnel: w293 -> [_ w304]
                frame False {
                  w299 = T2."Enabled" ("Disabled")
                  n231 = property on="Capture123" class="Bool (strict)"("Blinking"=FALSE) -> ()  [unwired: 2 in, 2 out]
                  n232 = property on="Tab Control" class="TabCtl (strict)"("PageSelVis"=TRUE ("Page Selector Visible")) -> ()  [unwired: 2 in, 2 out]
                  n233 = property on="Clear123" class="Bool"("DisabledEnum"=w299) -> ()  [unwired: 2 in, 2 out]
                  n234 = property on="Samples Per Second" class="Knob (strict)"("DisabledEnum"=w299) -> ()  [unwired: 2 in, 2 out]
                  n235 = property on="Save123" class="Bool"("DisabledEnum"=w299) -> ()  [unwired: 2 in, 2 out]
                  n236 = property on="Print123" class="Bool"("DisabledEnum"=w299) -> ()  [unwired: 2 in, 2 out]
                  n237 = property on="Samples box123" class="Bool"("DisabledEnum"=w299) -> ()  [unwired: 2 in, 2 out]
                  n238 = property on="stop" class="Bool (strict)"("DisabledEnum"=w299) -> ()  [unwired: 2 in, 2 out]
                }
                frame True {
                  w302 = T2."Disabled and Grayed Out" ("Disabled")
                  w311 = 10106 items=["default"=-1, "RSE"=10083, "NRSE"=10078, "Differential"=10106, "Pseudodifferential"=12529] ("input terminal configuration")
                  w314 = T22 0 items=["no dialog", "OK message", "continue or stop message", "OK message + warnings", "continue/stop + warnings"] ("type of dialog (OK msg:1)")
                  n239 = property on="Save123" class="Bool"("DisabledEnum"=w302) -> ()  [unwired: 2 in, 2 out]
                  n240 = property on="Samples box123" class="Bool"("DisabledEnum"=w302) -> ()  [unwired: 2 in, 2 out]
                  n241 = property on="stop" class="Bool (strict)"("DisabledEnum"=w302) -> ()  [unwired: 2 in, 2 out]
                  n242 = call-poly <vilib>:"DAQmx Create Virtual Channel.vi"("input terminal configuration"=w311, "physical channels"=w304) -> ("task out"=w321:refnum<k21>, "error out"=w319:errorcluster)  [unwired: 12 in]
                  n243 = property on="Tab Control" class="TabCtl (strict)"("PageSelVis"=FALSE ("Page Selector Visible")) -> ()  [unwired: 2 in, 2 out]
                  n244 = Divide(x=1000.0, y="Samples Per Second") -> (x/y=w303:dbl)
                  n245 = call-poly <vilib>:"DAQmx Timing.vi"("task/channels in"=w321, "samples per channel"=100000, "rate"="Samples Per Second", "error in"=w319) -> ("task out"=w320:refnum<k21>, "error out"=w318:errorcluster)  [unwired: 10 in]
                  n246 = node-c288(w303) -> (w309:T4)
                  n247 = property on="Capture123" class="Bool (strict)"("Blinking"=TRUE) -> ()  [unwired: 2 in, 2 out]
                  n248 = property on="Clear123" class="Bool"("DisabledEnum"=w302) -> ()  [unwired: 2 in, 2 out]
                  n249 = property on="Samples Per Second" class="Knob (strict)"("DisabledEnum"=w302) -> ()  [unwired: 2 in, 2 out]
                  n250 = property on="Print123" class="Bool"("DisabledEnum"=w302) -> ()  [unwired: 2 in, 2 out]
                  n251 = property on="Samples Per Second" class="Knob (strict)"("DisabledEnum"=w302) -> ()  [unwired: 2 in, 2 out]
                  n252 = call <vilib>:"DAQmx Start Task.vi"("task/channels in"=w320, "error in"=w318) -> ("task out"=w317:refnum<k21>, "error out"=w316:errorcluster)  [unwired: 12 in]
                  n253 = timed-loop {
                    tunnel: w317 -> [w341]
                    tunnel: w316 -> [w340]
                    tunnel: [w339] -> w313
                    tunnel: [w338] -> w312
                    timing: w309 -> [_]
                    timing-out: [_] -> w308
                    tunnel: w303 -> [w327]
                    stop <- w330 stop-if-true
                    n254 = node-c288() -> ()  [unwired: 1 in]
                    n255 = call-poly <vilib>:"DAQmx Read.vi"("task/channels in"=w341, "number of samples per channel"=1, "error in"=w340) -> ("task out"=w339:refnum<k21>, "data"=w336:waveform(dbl)[], "error out"=w338:errorcluster)  [unwired: 10 in]
                    n256 = Get Date/Time In Seconds() -> (seconds since 1Jan1904=w326:timestamp)
                    n257 = Split Signals(w336) -> (w333:dynamicdata, w335:dynamicdata, w325:dynamicdata)  [unwired: 3 in]
                    n258 = call "Convert from Dynamic Data9"("Dynamic Data Type"=w333) -> ("Array"=w332:dbl[])  [unwired: 3 in]
                    n259 = call "Convert from Dynamic Data5"("Dynamic Data Type"=w335) -> ("Array"=w334:dbl[])  [unwired: 3 in]
                    n260 = call "Convert from Dynamic Data12"("Dynamic Data Type"=w325) -> ("Array"=w324:dbl[])  [unwired: 3 in]
                    n261 = local read "Capture123"() -> (w329:bool)
                    n262 = Bundle By Name("Y"=w332, "t0"=w326, "dt"=w327) -> (w331:waveform(dbl))  [unwired: 1 in]
                    n263 = Bundle By Name("Y"=w334, "t0"=w326, "dt"=w327) -> (w328:waveform(dbl))  [unwired: 1 in]
                    n264 = Bundle By Name("Y"=w324, "t0"=w326, "dt"=w327) -> (w323:waveform(dbl))  [unwired: 1 in]
                    n265 = Merge Signals(w331, w328, w323) -> (→"Waveform Chart123":dynamicdata)
                    n266 = node-c288() -> ()  [unwired: 1 in, 1 out]
                    n267 = Not(x=w329) -> (.not. x?=w330:bool)
                  }
                  n268 = node-c288(w308) -> ()  [unwired: 1 out]
                  n269 = call <vilib>:"DAQmx Clear Task.vi"("task in"=w313, "error in"=w312) -> ("error out"=w315:errorcluster)  [unwired: 13 in]
                  n270 = call <vilib>:"Simple Error Handler.vi"("type of dialog (OK msg:1)"=w314, "error in (no error)"=w315) -> ()  [unwired: 3 in, 5 out]
                }
              }
            }
            event "Print123": Value Change {
              n271 = event-data() -> ()  [unwired: 1 in, 5 out]
              n272 = case shown="True" "Print123" {
                frame False {
                }
                frame True {
                  w350 = T22 0 items=["no dialog", "OK message", "continue or stop message", "OK message + warnings", "continue/stop + warnings"] ("type of dialog (OK msg:1)")
                  w354 = T24 1 items=["Complete front panel", "Visible portion of front panel", "Icon, description, panel and diagram", "Documentation: Using the panel", "Documentation: Using as a subVI", "Documentation: Complete", "Documentation: Custom"] ("contents (complete front panel)")
                  n273 = call-poly <vilib>:"Easy Print VI Panel or Documentation.vi"("custom contents options"=T20 {"include VI connector and icon"=FALSE, "include VI description"=FALSE, "include front panel"=FALSE, "surround front panel with border"=FALSE, "list of controls options"={"include list of controls"=FALSE, "list which controls?"=0, "include control descriptions?"=FALSE, "include control data types?"=FALSE}, "block diagram options"={"include block diagram"=FALSE, "hidden frames"=FALSE, "ordered (repeat from higher level if nested)"=FALSE}, "include VI hierarchy"=FALSE, "include list of subVIs"=FALSE, "include VI history"=FALSE, "include Express VI configuration information"=FALSE}, "layout options"=T8 {"orientation (unchanged)"=2, "panel scaling for page (unchanged)"=2, "margins"={"override VI margins (false)"=FALSE, "margins (1.00)"={"top"=1.0, "left"=1.0, "right"=1.0, "bottom"=1.0}, "measurement system (default)"=0}, "printer options"={"destination printer name (current)"="", "printing method (unchanged)"=0, "color or monochrome (unchanged)"=0}, "page header options"={"page headers (unchanged)"=1, "page header content options"={"Include VI Name"=TRUE, "Include VI Path"=TRUE, "Include Last Modification Date"=TRUE, "Include Date Printed"=TRUE, "Include Page Number"=TRUE, "Include VI Icon"=TRUE}}}, "contents (complete front panel)"=w354) -> ("error out"=w351:errorcluster)  [unwired: 3 in, 5 out]
                  n274 = call <vilib>:"Simple Error Handler.vi"("type of dialog (OK msg:1)"=w350, "error in (no error)"=w351) -> ("error?"=w349:bool)  [unwired: 3 in, 4 out]
                  n275 = case shown="True" w349 {
                    tunnel: [w355 _] -> _
                    tunnel: [_ w356] -> _
                    frame False {
                      n276 = call "Display Message to User7"() -> ("OK"=w355:bool)  [unwired: 10 in, 1 out]
                    }
                    frame True {
                      n277 = call "Display Message to User8"() -> ("OK"=w356:bool)  [unwired: 10 in, 1 out]
                    }
                  }
                }
              }
            }
            event "Clear123": Value Change {
              n278 = event-data() -> ()  [unwired: 1 in, 5 out]
              n279 = case shown="True" "Clear123" {
                frame False {
                }
                frame True {
                  n280 = invoke on="Waveform Chart123" class="WFChart (strict)" method="Reinit To Default"() -> ()  [unwired: 3 in, 3 out]
                  n281 = property on="Waveform Chart123" class="WFChart (strict)"("History Data"=dynamicdata[] []) -> ()  [unwired: 2 in, 2 out]
                }
              }
            }
            event "Save123": Value Change {
              n282 = event-data() -> ()  [unwired: 1 in, 5 out]
              n283 = case shown="True" "Save123" {
                frame False {
                }
                frame True {
                  w360 = T22 0 items=["no dialog", "OK message", "continue or stop message", "OK message + warnings", "continue/stop + warnings"] ("type of dialog (OK msg:1)")
                  n284 = call "File Dialog3"("prompt"="FIle to save to", "pattern (all files)"="*.txt", "pattern label"="Text File") -> ("selected path"=w364:path, "exists"=w362:bool, "cancelled"=w363:bool, "error out"=w361:errorcluster)  [unwired: 9 in]
                  n285 = call <vilib>:"Simple Error Handler.vi"("type of dialog (OK msg:1)"=w360, "error in (no error)"=w361) -> ()  [unwired: 3 in, 5 out]
                  n286 = case shown="False" w363 {
                    tunnel: w364 -> [w370 _]
                    tunnel: w362 -> [w371 _]
                    frame False {
                      n287 = case shown="True" w371 {
                        tunnel: w370 -> [w421 w424]
                        tunnel: [TRUE w423] -> w369
                        tunnel: [w421 w424] -> w368
                        frame False {
                        }
                        frame True {
                          n288 = Two Button Dialog(message="File exists - Overwrite?") -> (T button?=w423:bool)  [unwired: 2 in]
                        }
                      }
                      n289 = case shown="True" w369 {
                        tunnel: w368 -> [_ w396]
                        frame False {
                        }
                        frame True {
                          w373 = "\t"
                          w383 = T23 2 items=["both", "start of string", "end of string"] ("location (both)")
                          w374 = "\r\n"
                          n290 = property on="Waveform Chart123" class="WFChart (strict)"() -> ("History Data"=w379:dynamicdata[])  [unwired: 2 in, 2 out]
                          n291 = Get Date/Time In Seconds() -> (seconds since 1Jan1904=w387:timestamp)
                          n292 = for {
                            tunnel: w379 -> [w404] mode=indexing
                            tunnel: [w407] -> w375 mode=indexing
                            w400 = i16 6 ("width (-)")
                            n293 = call "Convert from Dynamic Data10"("Dynamic Data Type"=w404) -> ("Array"=w406:dbl[][])  [unwired: 3 in]
                            n294 = call "Convert from Dynamic Data11"("Dynamic Data Type"=w404) -> ("Waveform"=w403:waveform(dbl))  [unwired: 3 in]
                            n295 = Unbundle By Name(w403) -> ("t0"=w402:timestamp)
                            n296 = Reshape Array(w406, 4 ("dimension size")) -> (w419:dbl[])
                            n297 = Rotate 1D Array(1:w419, 2:1 ("n")) -> (0:w397:dbl[])
                            n298 = Format Date/Time String(time format string (%c)="%H:%M:%S%3u", seconds (now)=w402) -> (date/time string=w405:string)  [unwired: 1 in]
                            n299 = Index Array(array=w397, index=0) -> ()  [unwired: 1 out]
                            n300 = Index Array(array=w397, index=1) -> (element=w413:dbl)
                            n301 = Index Array(array=w397, index=2) -> (element=w412:dbl)
                            n302 = Index Array(array=w397, index=3) -> (element=w399:dbl)
                            n303 = Number To Fractional String(number=w413, precision (6)=w400) -> (F-format string=w410:string)  [unwired: 2 in]
                            n304 = Number To Fractional String(number=w412, precision (6)=w400) -> (F-format string=w411:string)  [unwired: 2 in]
                            n305 = Number To Fractional String(number=w399, precision (6)=w400) -> (F-format string=w398:string)  [unwired: 2 in]
                            n306 = Build Array(w410, w410, w411, w398) -> (w409:string[])
                            n307 = Replace Array Subset(array=w409, new element=w405, index=0) -> (w407:string[])
                          }
                          n308 = Get Date/Time String(date format (0)=enum16{"short", "long", "abbreviated"}."abbreviated", seconds (now)=w387) -> (date string=w389:string, time string=w390:string)  [unwired: 1 in]
                          n309 = call <vilib>:"Space Constant.vi"() -> ("String"=w384:string)
                          n310 = Concatenate Strings("Chart Recorder Data File" ("HeaderTxtIn"), w384, w389, w384, w390, w374, "Time (s)", w373, "CH1 (V)  ", w373, "CH2 (V)  ", w373, "CH3 (V)  ", w374) -> (w381:string)
                          n311 = Open/Create/Replace File(file path (use dialog)=w396, operation (0:open)=T7."replace or create", access (0:read/write)=enum16{"read/write", "read-only", "write-only"}."write-only") -> (refnum out=w395:refnum<file>)  [unwired: 3 in, 2 out]
                          n312 = Write to Text File(file (use dialog)=w395, text=w381) -> (refnum out=w391:refnum<file>)  [unwired: 2 in, 2 out]
                          n313 = Array To Spreadsheet String(array=w375, 3:"%.12f" ("format string")) -> (spreadsheet string=w377:string)  [unwired: 1 in]
                          n314 = call <vilib>:"Trim Whitespace.vi"("string"=w377, "location (both)"=w383) -> ("trimmed string"=w382:string)
                          n315 = Write to Text File(file (use dialog)=w391, text=w382) -> (refnum out=w392:refnum<file>)  [unwired: 2 in, 2 out]
                          n316 = Close File(refnum=w392) -> ()  [unwired: 1 in, 2 out]
                        }
                      }
                    }
                    frame True {
                    }
                  }
                }
              }
            }
          }
          n317 = local read "stop"() -> (w286:bool)
          n318 = property on="Tab Control" class="TabCtl (strict)"() -> ("Value"=w289:T1)  [unwired: 2 in, 2 out]
          n319 = Not Equal?(x=w289, y=T3."CH1+CH2+CH3 vs. Time" ("Tab Control")) -> (x != y?=w288:bool)
          n320 = Or(x=w286, y=w288) -> (x .or. y?=w287:bool)
        }
      }
      frame "CH1+CH2+CH3+CH4 vs. Time" {
        n321 = while {
          tunnel: [w427] -> w426
          stop <- w428 stop-if-true
          n322 = event shown="[1] \"Capture1234\": Value Change" {
            selector: _ -> [_ _ _ _ _]
            dyn-events: _ -> [_ _ _ _ _]
            timeout: 10 -> [_ _ _ _ _]
            event Timeout {
              n323 = event-data() -> ()  [unwired: 1 in, 2 out]
            }
            event "Capture1234": Value Change {
              n324 = event-data() -> ()  [unwired: 1 in, 1 out]
              n325 = property class="DAQmx System"() -> ("DevNames"=w435:tag[])  [unwired: 2 in, 2 out]
              n326 = Index Array(array=w435, index=0) -> (element=w438:tag)
              n327 = Concatenate Strings(w438, "/ai0:3" ("string")) -> (w434:string)
              n328 = case shown="False" "Capture1234" {
                tunnel: w434 -> [_ w445]
                frame False {
                  w440 = T2."Enabled" ("Disabled")
                  n329 = property on="Capture1234" class="Bool (strict)"("Blinking"=FALSE) -> ()  [unwired: 2 in, 2 out]
                  n330 = property on="Clear1234" class="Bool"("DisabledEnum"=w440) -> ()  [unwired: 2 in, 2 out]
                  n331 = property on="Samples Per Second" class="Knob (strict)"("DisabledEnum"=w440) -> ()  [unwired: 2 in, 2 out]
                  n332 = property on="Save1234" class="Bool"("DisabledEnum"=w440) -> ()  [unwired: 2 in, 2 out]
                  n333 = property on="Tab Control" class="TabCtl (strict)"("PageSelVis"=TRUE ("Page Selector Visible")) -> ()  [unwired: 2 in, 2 out]
                  n334 = property on="stop" class="Bool (strict)"("DisabledEnum"=w440) -> ()  [unwired: 2 in, 2 out]
                  n335 = property on="Print1234" class="Bool"("DisabledEnum"=w440) -> ()  [unwired: 2 in, 2 out]
                  n336 = property on="Samples box1234" class="Bool"("DisabledEnum"=w440) -> ()  [unwired: 2 in, 2 out]
                }
                frame True {
                  w443 = T2."Disabled and Grayed Out" ("Disabled")
                  w452 = 10106 items=["default"=-1, "RSE"=10083, "NRSE"=10078, "Differential"=10106, "Pseudodifferential"=12529] ("input terminal configuration")
                  w455 = T22 0 items=["no dialog", "OK message", "continue or stop message", "OK message + warnings", "continue/stop + warnings"] ("type of dialog (OK msg:1)")
                  n337 = property on="Samples box1234" class="Bool"("DisabledEnum"=w443) -> ()  [unwired: 2 in, 2 out]
                  n338 = property on="stop" class="Bool (strict)"("DisabledEnum"=w443) -> ()  [unwired: 2 in, 2 out]
                  n339 = property on="Save1234" class="Bool"("DisabledEnum"=w443) -> ()  [unwired: 2 in, 2 out]
                  n340 = call-poly <vilib>:"DAQmx Create Virtual Channel.vi"("input terminal configuration"=w452, "physical channels"=w445) -> ("task out"=w462:refnum<k21>, "error out"=w460:errorcluster)  [unwired: 12 in]
                  n341 = property on="Tab Control" class="TabCtl (strict)"("PageSelVis"=FALSE ("Page Selector Visible")) -> ()  [unwired: 2 in, 2 out]
                  n342 = Divide(x=1000.0, y="Samples Per Second") -> (x/y=w444:dbl)
                  n343 = call-poly <vilib>:"DAQmx Timing.vi"("task/channels in"=w462, "samples per channel"=100000, "rate"="Samples Per Second", "error in"=w460) -> ("task out"=w461:refnum<k21>, "error out"=w459:errorcluster)  [unwired: 10 in]
                  n344 = node-c288(w444) -> (w450:T4)
                  n345 = property on="Capture1234" class="Bool (strict)"("Blinking"=TRUE) -> ()  [unwired: 2 in, 2 out]
                  n346 = property on="Clear1234" class="Bool"("DisabledEnum"=w443) -> ()  [unwired: 2 in, 2 out]
                  n347 = property on="Samples Per Second" class="Knob (strict)"("DisabledEnum"=w443) -> ()  [unwired: 2 in, 2 out]
                  n348 = property on="Print1234" class="Bool"("DisabledEnum"=w443) -> ()  [unwired: 2 in, 2 out]
                  n349 = property on="Samples Per Second" class="Knob (strict)"("DisabledEnum"=w443) -> ()  [unwired: 2 in, 2 out]
                  n350 = call <vilib>:"DAQmx Start Task.vi"("task/channels in"=w461, "error in"=w459) -> ("task out"=w458:refnum<k21>, "error out"=w457:errorcluster)  [unwired: 12 in]
                  n351 = timed-loop {
                    tunnel: w458 -> [w485]
                    tunnel: w457 -> [w484]
                    tunnel: [w483] -> w454
                    tunnel: [w482] -> w453
                    timing: w450 -> [_]
                    timing-out: [_] -> w449
                    tunnel: w444 -> [w467]
                    stop <- w474 stop-if-true
                    n352 = node-c288() -> ()  [unwired: 1 in]
                    n353 = Get Date/Time In Seconds() -> (seconds since 1Jan1904=w466:timestamp)
                    n354 = call-poly <vilib>:"DAQmx Read.vi"("task/channels in"=w485, "number of samples per channel"=1, "error in"=w484) -> ("task out"=w483:refnum<k21>, "data"=w480:waveform(dbl)[], "error out"=w482:errorcluster)  [unwired: 10 in]
                    n355 = Split Signals(w480) -> (w477:dynamicdata, w479:dynamicdata, w471:dynamicdata, w465:dynamicdata)  [unwired: 4 in]
                    n356 = call "Convert from Dynamic Data14"("Dynamic Data Type"=w477) -> ("Array"=w476:dbl[])  [unwired: 3 in]
                    n357 = call "Convert from Dynamic Data13"("Dynamic Data Type"=w479) -> ("Array"=w478:dbl[])  [unwired: 3 in]
                    n358 = call "Convert from Dynamic Data15"("Dynamic Data Type"=w471) -> ("Array"=w470:dbl[])  [unwired: 3 in]
                    n359 = call "Convert from Dynamic Data18"("Dynamic Data Type"=w465) -> ("Array"=w464:dbl[])  [unwired: 3 in]
                    n360 = local read "Capture1234"() -> (w473:bool)
                    n361 = Bundle By Name("Y"=w476, "t0"=w466, "dt"=w467) -> (w475:waveform(dbl))  [unwired: 1 in]
                    n362 = Bundle By Name("Y"=w478, "t0"=w466, "dt"=w467) -> (w472:waveform(dbl))  [unwired: 1 in]
                    n363 = Bundle By Name("Y"=w470, "t0"=w466, "dt"=w467) -> (w468:waveform(dbl))  [unwired: 1 in]
                    n364 = Bundle By Name("Y"=w464, "t0"=w466, "dt"=w467) -> (w463:waveform(dbl))  [unwired: 1 in]
                    n365 = node-c288() -> ()  [unwired: 1 in, 1 out]
                    n366 = Merge Signals(w475, w472, w468, w463) -> (→"Waveform Chart1234":dynamicdata)
                    n367 = Not(x=w473) -> (.not. x?=w474:bool)
                  }
                  n368 = node-c288(w449) -> ()  [unwired: 1 out]
                  n369 = call <vilib>:"DAQmx Clear Task.vi"("task in"=w454, "error in"=w453) -> ("error out"=w456:errorcluster)  [unwired: 13 in]
                  n370 = call <vilib>:"Simple Error Handler.vi"("type of dialog (OK msg:1)"=w455, "error in (no error)"=w456) -> ()  [unwired: 3 in, 5 out]
                }
              }
            }
            event "Print1234": Value Change {
              n371 = event-data() -> ()  [unwired: 1 in, 5 out]
              n372 = case shown="True" "Print1234" {
                frame False {
                }
                frame True {
                  w494 = T22 0 items=["no dialog", "OK message", "continue or stop message", "OK message + warnings", "continue/stop + warnings"] ("type of dialog (OK msg:1)")
                  w498 = T24 1 items=["Complete front panel", "Visible portion of front panel", "Icon, description, panel and diagram", "Documentation: Using the panel", "Documentation: Using as a subVI", "Documentation: Complete", "Documentation: Custom"] ("contents (complete front panel)")
                  n373 = call-poly <vilib>:"Easy Print VI Panel or Documentation.vi"("custom contents options"=T20 {"include VI connector and icon"=FALSE, "include VI description"=FALSE, "include front panel"=FALSE, "surround front panel with border"=FALSE, "list of controls options"={"include list of controls"=FALSE, "list which controls?"=0, "include control descriptions?"=FALSE, "include control data types?"=FALSE}, "block diagram options"={"include block diagram"=FALSE, "hidden frames"=FALSE, "ordered (repeat from higher level if nested)"=FALSE}, "include VI hierarchy"=FALSE, "include list of subVIs"=FALSE, "include VI history"=FALSE, "include Express VI configuration information"=FALSE}, "layout options"=T8 {"orientation (unchanged)"=2, "panel scaling for page (unchanged)"=2, "margins"={"override VI margins (false)"=FALSE, "margins (1.00)"={"top"=1.0, "left"=1.0, "right"=1.0, "bottom"=1.0}, "measurement system (default)"=0}, "printer options"={"destination printer name (current)"="", "printing method (unchanged)"=0, "color or monochrome (unchanged)"=0}, "page header options"={"page headers (unchanged)"=1, "page header content options"={"Include VI Name"=TRUE, "Include VI Path"=TRUE, "Include Last Modification Date"=TRUE, "Include Date Printed"=TRUE, "Include Page Number"=TRUE, "Include VI Icon"=TRUE}}}, "contents (complete front panel)"=w498) -> ("error out"=w495:errorcluster)  [unwired: 3 in, 5 out]
                  n374 = call <vilib>:"Simple Error Handler.vi"("type of dialog (OK msg:1)"=w494, "error in (no error)"=w495) -> ("error?"=w493:bool)  [unwired: 3 in, 4 out]
                  n375 = case shown="True" w493 {
                    tunnel: [w499 _] -> _
                    tunnel: [_ w500] -> _
                    frame False {
                      n376 = call "Display Message to User9"() -> ("OK"=w499:bool)  [unwired: 10 in, 1 out]
                    }
                    frame True {
                      n377 = call "Display Message to User10"() -> ("OK"=w500:bool)  [unwired: 10 in, 1 out]
                    }
                  }
                }
              }
            }
            event "Clear1234": Value Change {
              n378 = event-data() -> ()  [unwired: 1 in, 5 out]
              n379 = case shown="True" "Clear1234" {
                frame False {
                }
                frame True {
                  n380 = invoke on="Waveform Chart1234" class="WFChart (strict)" method="Reinit To Default"() -> ()  [unwired: 3 in, 3 out]
                  n381 = property on="Waveform Chart1234" class="WFChart (strict)"("History Data"=dynamicdata[] []) -> ()  [unwired: 2 in, 2 out]
                }
              }
            }
            event "Save1234": Value Change {
              n382 = event-data() -> ()  [unwired: 1 in, 5 out]
              n383 = case shown="True" "Save1234" {
                frame False {
                }
                frame True {
                  w504 = T22 0 items=["no dialog", "OK message", "continue or stop message", "OK message + warnings", "continue/stop + warnings"] ("type of dialog (OK msg:1)")
                  n384 = call "File Dialog4"("prompt"="FIle to save to", "pattern (all files)"="*.txt", "pattern label"="Text File") -> ("selected path"=w508:path, "exists"=w506:bool, "cancelled"=w507:bool, "error out"=w505:errorcluster)  [unwired: 9 in]
                  n385 = call <vilib>:"Simple Error Handler.vi"("type of dialog (OK msg:1)"=w504, "error in (no error)"=w505) -> ()  [unwired: 3 in, 5 out]
                  n386 = case shown="False" w507 {
                    tunnel: w508 -> [w514 _]
                    tunnel: w506 -> [w515 _]
                    frame False {
                      n387 = case shown="True" w515 {
                        tunnel: w514 -> [w569 w572]
                        tunnel: [TRUE w571] -> w513
                        tunnel: [w569 w572] -> w512
                        frame False {
                        }
                        frame True {
                          n388 = Two Button Dialog(message="File exists - Overwrite?") -> (T button?=w571:bool)  [unwired: 2 in]
                        }
                      }
                      n389 = case shown="True" w513 {
                        tunnel: w512 -> [_ w541]
                        frame False {
                        }
                        frame True {
                          w518 = "\t"
                          w528 = T23 2 items=["both", "start of string", "end of string"] ("location (both)")
                          w520 = "\r\n"
                          n390 = property on="Waveform Chart1234" class="WFChart (strict)"() -> ("History Data"=w524:dynamicdata[])  [unwired: 2 in, 2 out]
                          n391 = Get Date/Time In Seconds() -> (seconds since 1Jan1904=w532:timestamp)
                          n392 = for {
                            tunnel: w524 -> [w552] mode=indexing
                            tunnel: [w555] -> w521 mode=indexing
                            w547 = i16 6 ("width (-)")
                            n393 = call "Convert from Dynamic Data16"("Dynamic Data Type"=w552) -> ("Array"=w554:dbl[][])  [unwired: 3 in]
                            n394 = call "Convert from Dynamic Data17"("Dynamic Data Type"=w552) -> ("Waveform"=w551:waveform(dbl))  [unwired: 3 in]
                            n395 = Unbundle By Name(w551) -> ("t0"=w550:timestamp)
                            n396 = Reshape Array(w554, 5 ("dimension size")) -> (w567:dbl[])
                            n397 = Rotate 1D Array(1:w567, 2:1 ("n")) -> (0:w545:dbl[])
                            n398 = Format Date/Time String(time format string (%c)="%H:%M:%S%3u", seconds (now)=w550) -> (date/time string=w553:string)  [unwired: 1 in]
                            n399 = Index Array(array=w545, index=0) -> ()  [unwired: 1 out]
                            n400 = Index Array(array=w545, index=1) -> (element=w561:dbl)
                            n401 = Index Array(array=w545, index=2) -> (element=w560:dbl)
                            n402 = Index Array(array=w545, index=3) -> (element=w544:dbl)
                            n403 = Index Array(array=w545, index=4) -> (element=w546:dbl)
                            n404 = Number To Fractional String(number=w561, precision (6)=w547) -> (F-format string=w558:string)  [unwired: 2 in]
                            n405 = Number To Fractional String(number=w560, precision (6)=w547) -> (F-format string=w559:string)  [unwired: 2 in]
                            n406 = Number To Fractional String(number=w544, precision (6)=w547) -> (F-format string=w543:string)  [unwired: 2 in]
                            n407 = Number To Fractional String(number=w546, precision (6)=w547) -> (F-format string=w542:string)  [unwired: 2 in]
                            n408 = Build Array(w558, w558, w559, w543, w542) -> (w557:string[])
                            n409 = Replace Array Subset(array=w557, new element=w553, index=0) -> (w555:string[])
                          }
                          n410 = Get Date/Time String(date format (0)=enum16{"short", "long", "abbreviated"}."abbreviated", seconds (now)=w532) -> (date string=w534:string, time string=w535:string)  [unwired: 1 in]
                          n411 = call <vilib>:"Space Constant.vi"() -> ("String"=w529:string)
                          n412 = Concatenate Strings("Chart Recorder Data File" ("HeaderTxtIn"), w529, w534, w529, w535, w520, "Time (s)", w518, "CH1 (V)  ", w518, "CH2 (V)  ", w518, "CH3 (V)  ", w518, "CH4 (V)  ", w520) -> (w526:string)
                          n413 = Open/Create/Replace File(file path (use dialog)=w541, operation (0:open)=T7."replace or create", access (0:read/write)=enum16{"read/write", "read-only", "write-only"}."write-only") -> (refnum out=w540:refnum<file>)  [unwired: 3 in, 2 out]
                          n414 = Write to Text File(file (use dialog)=w540, text=w526) -> (refnum out=w536:refnum<file>)  [unwired: 2 in, 2 out]
                          n415 = Array To Spreadsheet String(array=w521, 3:"%.12f" ("format string")) -> (spreadsheet string=w523:string)  [unwired: 1 in]
                          n416 = call <vilib>:"Trim Whitespace.vi"("string"=w523, "location (both)"=w528) -> ("trimmed string"=w527:string)
                          n417 = Write to Text File(file (use dialog)=w536, text=w527) -> (refnum out=w537:refnum<file>)  [unwired: 2 in, 2 out]
                          n418 = Close File(refnum=w537) -> ()  [unwired: 1 in, 2 out]
                        }
                      }
                    }
                    frame True {
                    }
                  }
                }
              }
            }
          }
          n419 = local read "stop"() -> (w427:bool)
          n420 = property on="Tab Control" class="TabCtl (strict)"() -> ("Value"=w431:T1)  [unwired: 2 in, 2 out]
          n421 = Not Equal?(x=w431, y=T3."CH1+CH2+CH3+CH4 vs. Time" ("Tab Control")) -> (x != y?=w429:bool)
          n422 = Or(x=w427, y=w429) -> (x .or. y?=w428:bool)
        }
      }
      frame "CH1 vs. CH2 " {
        n423 = while {
          tunnel: [w577] -> w574
          stop <- w578 stop-if-true
          n424 = event shown="[1] \"Capture1v2\": Value Change" {
            selector: _ -> [_ _ _ _ _]
            dyn-events: _ -> [_ _ _ _ _]
            timeout: 10 -> [_ _ _ _ _]
            event Timeout {
              n425 = event-data() -> ()  [unwired: 1 in, 2 out]
            }
            event "Capture1v2": Value Change {
              n426 = event-data() -> ()  [unwired: 1 in, 1 out]
              n427 = property class="DAQmx System"() -> ("DevNames"=w583:tag[])  [unwired: 2 in, 2 out]
              n428 = Index Array(array=w583, index=0) -> (element=w586:tag)
              n429 = Concatenate Strings(w586, "/ai0:1" ("string")) -> (w582:string)
              n430 = case shown="True" "Capture1v2" {
                tunnel: w582 -> [_ w604]
                frame False {
                  w588 = T2."Enabled" ("Disabled")
                  n431 = property on="Tab Control" class="TabCtl (strict)"("PageSelVis"=TRUE ("Page Selector Visible")) -> ()  [unwired: 2 in, 2 out]
                  n432 = property on="Capture1v2" class="Bool (strict)"("Blinking"=FALSE) -> ()  [unwired: 2 in, 2 out]
                  n433 = property on="Samples box1v2" class="Bool"("DisabledEnum"=w588) -> ()  [unwired: 2 in, 2 out]
                  n434 = property on="Samples Per Second" class="Knob (strict)"("DisabledEnum"=w588) -> ()  [unwired: 2 in, 2 out]
                  n435 = property on="Print1v2" class="Bool"("DisabledEnum"=w588) -> ()  [unwired: 2 in, 2 out]
                  n436 = property on="Save1v2" class="Bool"("DisabledEnum"=w588) -> ()  [unwired: 2 in, 2 out]
                  n437 = property on="stop" class="Bool (strict)"("DisabledEnum"=w588) -> ()  [unwired: 2 in, 2 out]
                  n438 = property on="Clear1v2" class="Bool"("DisabledEnum"=w588) -> ()  [unwired: 2 in, 2 out]
                }
                frame True {
                  w590 = 10123 items=["Finite Samples"=10178, "Continuous Samples"=10123, "Hardware Timed Single Point"=12522] ("sample mode")
                  w592 = T2."Disabled and Grayed Out" ("Disabled")
                  w597 = T22 0 items=["no dialog", "OK message", "continue or stop message", "OK message + warnings", "continue/stop + warnings"] ("type of dialog (OK msg:1)")
                  n439 = property on="Tab Control" class="TabCtl (strict)"("PageSelVis"=FALSE ("Page Selector Visible")) -> ()  [unwired: 2 in, 2 out]
                  n440 = call-poly <vilib>:"DAQmx Create Virtual Channel.vi"("physical channels"=w604) -> ("task out"=w602:refnum<k21>, "error out"=w606:errorcluster)  [unwired: 13 in]
                  n441 = property on="Capture1v2" class="Bool (strict)"("Blinking"=TRUE) -> ()  [unwired: 2 in, 2 out]
                  n442 = Divide(x=1000.0, y="Samples Per Second") -> (x/y=w594:dbl)
                  n443 = call-poly <vilib>:"DAQmx Timing.vi"("task/channels in"=w602, "sample mode"=w590, "rate"=100000.0, "error in"=w606) -> ("task out"=w601:refnum<k21>, "error out"=w605:errorcluster)  [unwired: 10 in]
                  n444 = node-c288(w594) -> (w610:T4)
                  n445 = property on="Samples box1v2" class="Bool"("DisabledEnum"=w592) -> ()  [unwired: 2 in, 2 out]
                  n446 = property on="Samples Per Second" class="Knob (strict)"("DisabledEnum"=w592) -> ()  [unwired: 2 in, 2 out]
                  n447 = property on="Print1v2" class="Bool"("DisabledEnum"=w592) -> ()  [unwired: 2 in, 2 out]
                  n448 = property on="Save1v2" class="Bool"("DisabledEnum"=w592) -> ()  [unwired: 2 in, 2 out]
                  n449 = property on="stop" class="Bool (strict)"("DisabledEnum"=w592) -> ()  [unwired: 2 in, 2 out]
                  n450 = property on="Clear1v2" class="Bool"("DisabledEnum"=w592) -> ()  [unwired: 2 in, 2 out]
                  n451 = call <vilib>:"DAQmx Start Task.vi"("task/channels in"=w601, "error in"=w605) -> ("task out"=w600:refnum<k21>, "error out"=w599:errorcluster)  [unwired: 12 in]
                  n452 = timed-loop {
                    timing: w610 -> [_]
                    timing-out: [_] -> w609
                    tunnel: w600 -> [w626]
                    tunnel: w599 -> [w625]
                    tunnel: [w622] -> w595
                    tunnel: [w624] -> w596
                    i -> [w616]
                    stop <- w613 stop-if-true
                    n453 = node-c288() -> ()  [unwired: 1 in, 1 out]
                    n454 = Equal To 0?(x=w616) -> (x = 0?=w618:bool)
                    n455 = call-poly <vilib>:"DAQmx Read.vi"("task/channels in"=w626, "number of samples per channel"=1, "error in"=w625) -> ("task out"=w622:refnum<k21>, "data"=w621:waveform(dbl)[], "error out"=w624:errorcluster)  [unwired: 10 in]
                    n456 = Select(t=w618, s="Reset", f=FALSE) -> (s? t:f=w615:bool)
                    n457 = Split Signals(w621) -> (w612:dynamicdata, w611:dynamicdata)  [unwired: 2 in]
                    n458 = local read "Capture1v2"() -> (w614:bool)
                    n459 = call "Build XY Graph"("Reset"=w615, "Y Input"=w611, "X Input"=w612) -> ("XY Graph"=→"XY Graph":cluster{"Y":dbl[], "Y":dbl[]}[])  [unwired: 2 in, 6 out]
                    n460 = node-c288() -> ()  [unwired: 1 in, 1 out]
                    n461 = Not(x=w614) -> (.not. x?=w613:bool)
                  }
                  n462 = node-c288(w609) -> ()  [unwired: 1 out]
                  n463 = call <vilib>:"DAQmx Clear Task.vi"("task in"=w595, "error in"=w596) -> ("error out"=w598:errorcluster)  [unwired: 13 in]
                  n464 = call <vilib>:"Simple Error Handler.vi"("type of dialog (OK msg:1)"=w597, "error in (no error)"=w598) -> ()  [unwired: 3 in, 5 out]
                }
              }
            }
            event "Save1v2": Value Change {
              n465 = event-data() -> ()  [unwired: 1 in, 5 out]
              n466 = case shown="True" "Save1v2" {
                frame False {
                }
                frame True {
                  w634 = T22 0 items=["no dialog", "OK message", "continue or stop message", "OK message + warnings", "continue/stop + warnings"] ("type of dialog (OK msg:1)")
                  n467 = call "File Dialog5"("prompt"="FIle to save to", "pattern (all files)"="*.txt", "pattern label"="Text File") -> ("selected path"=w638:path, "exists"=w636:bool, "cancelled"=w637:bool, "error out"=w635:errorcluster)  [unwired: 9 in]
                  n468 = call <vilib>:"Simple Error Handler.vi"("type of dialog (OK msg:1)"=w634, "error in (no error)"=w635) -> ()  [unwired: 3 in, 5 out]
                  n469 = case shown="False" w637 {
                    tunnel: w638 -> [w644 _]
                    tunnel: w636 -> [w645 _]
                    frame False {
                      n470 = case shown="True" w645 {
                        tunnel: w644 -> [w673 w676]
                        tunnel: [TRUE w675] -> w643
                        tunnel: [w673 w676] -> w642
                        frame False {
                        }
                        frame True {
                          n471 = Two Button Dialog(message="File exists - Overwrite?") -> (T button?=w675:bool)  [unwired: 2 in]
                        }
                      }
                      n472 = case shown="True" w643 {
                        tunnel: w642 -> [_ w672]
                        frame False {
                        }
                        frame True {
                          w661 = T23 2 items=["both", "start of string", "end of string"] ("location (both)")
                          w646 = "\r\n"
                          n473 = Get Date/Time In Seconds() -> (seconds since 1Jan1904=w663:timestamp)
                          n474 = Get Date/Time String(date format (0)=enum16{"short", "long", "abbreviated"}."abbreviated", seconds (now)=w663) -> (date string=w665:string, time string=w666:string)  [unwired: 1 in]
                          n475 = local read "XY Graph"() -> (w650:cluster{"Y":dbl[], "Y":dbl[]}[])
                          n476 = Index Array(array=w650) -> (element=w654:cluster{"Y":dbl[], "Y":dbl[]})  [unwired: 1 in]
                          n477 = call <vilib>:"Space Constant.vi"() -> ("String"=w662:string)
                          n478 = Unbundle(w654) -> ("Y"=w653:dbl[], "Y"=w652:dbl[])
                          n479 = Build Array(w653, w652) -> (w651:dbl[][])
                          n480 = Concatenate Strings("Chart Recorder Data File" ("HeaderTxtIn"), w662, w665, w662, w666, w646, "CH1 (V)  ", "\t", "CH2 (V)  ", w646) -> (w659:string)
                          n481 = Transpose 2D Array(2D array=w651) -> (transposed array=w649:dbl[][])
                          n482 = Open/Create/Replace File(file path (use dialog)=w672, operation (0:open)=T7."replace or create", access (0:read/write)=enum16{"read/write", "read-only", "write-only"}."write-only") -> (refnum out=w671:refnum<file>)  [unwired: 3 in, 2 out]
                          n483 = Write to Text File(file (use dialog)=w671, text=w659) -> (refnum out=w667:refnum<file>)  [unwired: 2 in, 2 out]
                          n484 = Array To Spreadsheet String(array=w649, 3:"%.9f" ("format string")) -> (spreadsheet string=w656:string)  [unwired: 1 in]
                          n485 = call <vilib>:"Trim Whitespace.vi"("string"=w656, "location (both)"=w661) -> ("trimmed string"=w660:string)
                          n486 = Write to Text File(file (use dialog)=w667, text=w660) -> (refnum out=w668:refnum<file>)  [unwired: 2 in, 2 out]
                          n487 = Close File(refnum=w668) -> ()  [unwired: 1 in, 2 out]
                        }
                      }
                    }
                    frame True {
                    }
                  }
                }
              }
            }
            event "Print1v2": Value Change {
              n488 = event-data() -> ()  [unwired: 1 in, 5 out]
              n489 = case shown="True" "Print1v2" {
                frame False {
                }
                frame True {
                  w680 = T22 0 items=["no dialog", "OK message", "continue or stop message", "OK message + warnings", "continue/stop + warnings"] ("type of dialog (OK msg:1)")
                  w684 = T24 1 items=["Complete front panel", "Visible portion of front panel", "Icon, description, panel and diagram", "Documentation: Using the panel", "Documentation: Using as a subVI", "Documentation: Complete", "Documentation: Custom"] ("contents (complete front panel)")
                  n490 = call-poly <vilib>:"Easy Print VI Panel or Documentation.vi"("custom contents options"=T20 {"include VI connector and icon"=FALSE, "include VI description"=FALSE, "include front panel"=FALSE, "surround front panel with border"=FALSE, "list of controls options"={"include list of controls"=FALSE, "list which controls?"=0, "include control descriptions?"=FALSE, "include control data types?"=FALSE}, "block diagram options"={"include block diagram"=FALSE, "hidden frames"=FALSE, "ordered (repeat from higher level if nested)"=FALSE}, "include VI hierarchy"=FALSE, "include list of subVIs"=FALSE, "include VI history"=FALSE, "include Express VI configuration information"=FALSE}, "layout options"=T8 {"orientation (unchanged)"=2, "panel scaling for page (unchanged)"=2, "margins"={"override VI margins (false)"=FALSE, "margins (1.00)"={"top"=1.0, "left"=1.0, "right"=1.0, "bottom"=1.0}, "measurement system (default)"=0}, "printer options"={"destination printer name (current)"="", "printing method (unchanged)"=0, "color or monochrome (unchanged)"=0}, "page header options"={"page headers (unchanged)"=1, "page header content options"={"Include VI Name"=TRUE, "Include VI Path"=TRUE, "Include Last Modification Date"=TRUE, "Include Date Printed"=TRUE, "Include Page Number"=TRUE, "Include VI Icon"=TRUE}}}, "contents (complete front panel)"=w684) -> ("error out"=w681:errorcluster)  [unwired: 3 in, 5 out]
                  n491 = call <vilib>:"Simple Error Handler.vi"("type of dialog (OK msg:1)"=w680, "error in (no error)"=w681) -> ("error?"=w679:bool)  [unwired: 3 in, 4 out]
                  n492 = case shown="True" w679 {
                    tunnel: [w685 _] -> _
                    tunnel: [_ w686] -> _
                    frame False {
                      n493 = call "Display Message to User"() -> ("OK"=w685:bool)  [unwired: 10 in, 1 out]
                    }
                    frame True {
                      n494 = call "Display Message to User2"() -> ("OK"=w686:bool)  [unwired: 10 in, 1 out]
                    }
                  }
                }
              }
            }
            event "Clear1v2": Value Change {
              n495 = event-data() -> ()  [unwired: 1 in, 5 out]
              n496 = case shown="True" "Clear1v2" {
                frame False {
                }
                frame True {
                  n497 = local write "Reset"(TRUE ("Reset")) -> ()
                  n498 = property on="XY Graph" class="XYGraph (strict)"("Value"=cluster{"Y":dbl[], "Y":dbl[]}[] [] ("XY Graph")) -> ()  [unwired: 2 in, 2 out]
                }
              }
            }
          }
          n499 = property on="Tab Control" class="TabCtl (strict)"() -> ("Value"=w580:T1)  [unwired: 2 in, 2 out]
          n500 = Not Equal?(x=w580, y=T3."CH1 vs. CH2  " ("Tab Control")) -> (x != y?=w579:bool)
          n501 = local read "stop"() -> (w577:bool)
          n502 = Or(x=w577, y=w579) -> (x .or. y?=w578:bool)
        }
      }
    }
  }
  n503 = case shown="True" w10 {
    selector: w10 -> [_ w691]
    frame False {
    }
    frame True {
      n504 = flat-sequence {
        tunnel: w691 -> [w692]
        tunnel: [w692] -> w690
        frame #0 {
          n505 = control-ref of="This VI"() -> (w693:refnum<vi>)
          n506 = invoke class="VI" method="FP.Close"(reference=w693) -> ()  [unwired: 2 in, 3 out]
        }
      }
      n507 = Quit LabVIEW(quit? (T)=w690) -> ()
    }
  }
